vi "ELeye_V3.vi"() -> ()   [LabVIEW 2018]
uses:
  Keithley_622x_LV_8/Keithley 622x LV 8.0/Utility/Typedefs/KE622x -- Instrument Type.ctl
  Keithley_622x_LV_8/Keithley 622x LV 8.0/Typedefs/KE622x -- On Off Control.ctl
  Keithley_622x_LV_8/Keithley 622x LV 8.0/Configure/Source/Typedefs/KE622x -- Current Level.ctl
  ke236/KE236.LLB/Keith 236 Operate/Standby.vi
  <vilib>/Instr/_visa.llb/VISA Configure Serial Port (Instr).vi
  <vilib>/Utility/file.llb/Write Delimited Spreadsheet (DBL).vi
  Keithley_622x_LV_8/Keithley 622x LV 8.0/Keithley 622x.lvlib
panel:
  in  "Interline Delay (s)":dbl
  in  "SMU GPIB address":string="16"
  out "1D values":dbl[](array[numeric]) format="%.2f"
  out "1D Data ready":bool caption="1D ready"
  out "2D Data ready":bool caption="2D ready"
  in  "Filaname":string
  out "Y scale":dbl[](array[numeric]) format="%.2f"
  out "X scale":dbl[](array[numeric]) format="%.2f"
  out "2D XY array":dbl[][](array[numeric])
  out "IV 1D Graph":T1(graph)
  out "Time Trace":dbl(graph)
  in  "Sample SMU?":bool caption="SMU"
  in  "Sample Current Source?":bool caption="Source I"
  in  "Sample Gate?":bool caption="Gate V"
  out "Error SMU":errorcluster
  in  "Save":bool
  in  "Save Path":path
  in  "Compliance Current Drain":dbl=1e-06 caption="Compliance (A)" min=-0.001 max=0.001 step=1e-09 format="%#_6e"
  in  "Start VdVg Sweep":bool
  out "SMU Device Ready":bool
  in  "Initialize SMU":bool
  in  "SMU Resource":refnum<visa-resource-name> caption="SMU"
  out "Drain Device Ready":bool
  in  "Initialize Drain Source":bool
  in  "Compliance Shutoff":bool
  out "Voltage-Current 2D Graph":dbl[][](graph)
  out "Gate Device Ready":bool
  in  "Initialize Gate Generator":bool
  in  "Start IdVg Sweep":bool
  out "Error Current":errorcluster
  in  "Current Resource":refnum<visa-resource-name> caption="Current Source"
  out "Present Time":dbl caption="Time (s)"
  in  "Start Drain Sweep":bool
  out "Voltage Gate Value":dbl
  out "Voltage Drain Value":dbl
  in  "Step Voltage Drain":dbl
  in  "End Voltage Drain":dbl=-0.1
  in  "Start Voltage Drain":dbl=-0.1
  in  "Start Gate Sweep":bool
  in  "Sampling Mode":u16(ring) items=["Source V/Measure I", "Source I/Measure V"]
  in  "Start Voltage Gate":dbl=-2.0 caption="Start"
  in  "End Voltage Gate":dbl=2.0 caption="End"
  in  "Step Voltage Gate":dbl=0.1 caption="Step"
  in  "Sampling Number":u32=10 caption="Samples Number"
  in  "Start Sampling":bool
  in  "Stop Measurements":bool
  in  "Start CC Sweep":bool
  in  "Start Current Drain":dbl=1e-06 min=-0.001 max=0.001 step=1e-09 format="%#.6e"
  in  "End Current Drain":dbl=1e-06 min=-0.001 max=0.001 step=1e-09 format="%#_6e"
  in  "Step Current Drain":dbl=1e-06 min=-0.001 max=0.001 step=1e-09
  in  "Compliance Voltage Drain":dbl=10.0 caption="Compliance (V)"
  out "Current Drain Value":dbl
  out "Current Gate Value":dbl
  in  "Integration Time":dbl=100.0 caption="Int. Time (s)" format="%#_1f"
  in  "OneWay Sweep":bool caption="OneWay"
  in  "Step Delay (s)":dbl
  in  "Exit program":bool
  out "Error Gate":errorcluster
  in  "Gate resource":refnum<visa-resource-name> caption="Gate Generator"
  # "Gate (V)"
  # "Drain (V)"
  # "Drain (A)"
  # "Drain"
  # "Gate"
  # "(A)"
  # "(V)"
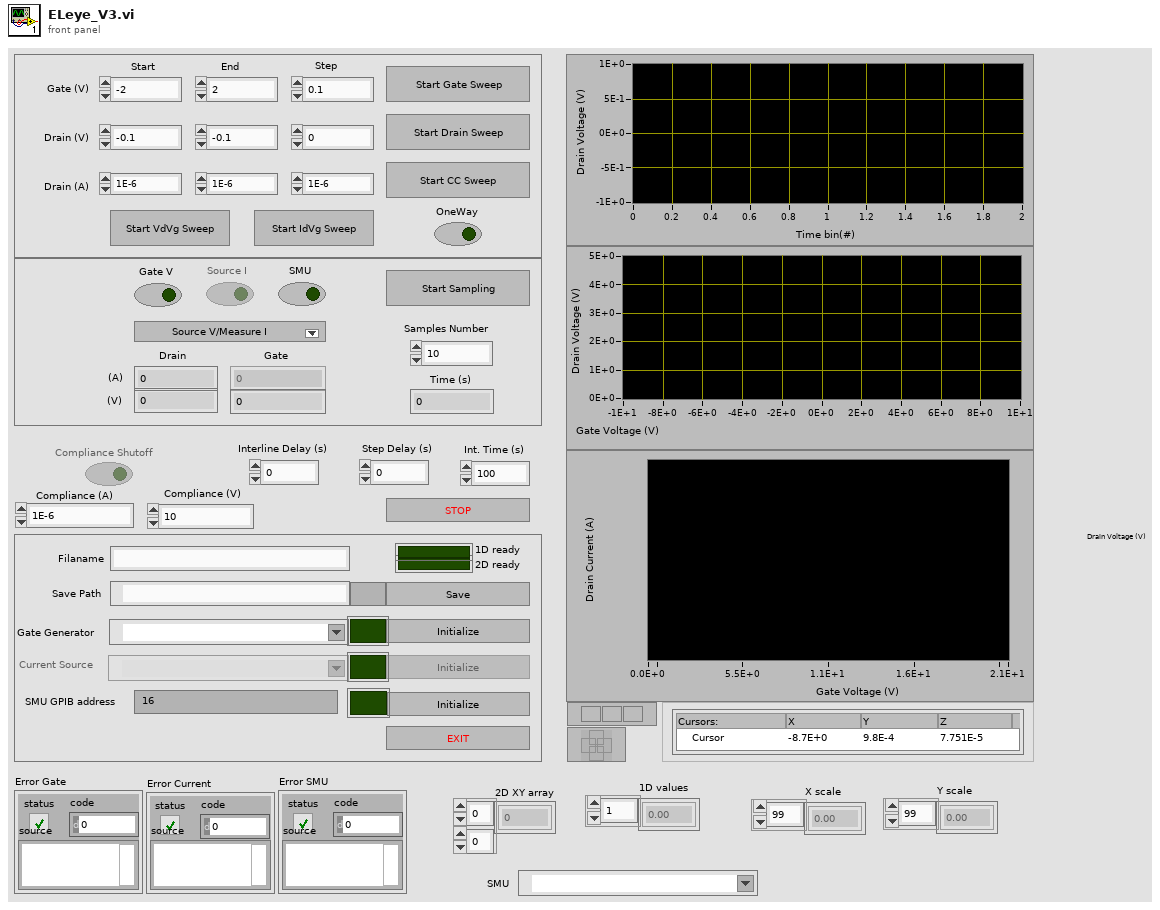
[diagram p1: front panel]
types:
  T1 = cluster{"Calibrated Array":dbl[], "Array F32":sgl[]}
  T2 = typedef "Keithley 622x.lvlib/KE622x -- On Off Control.ctl" = enum16{"Off", "On"}
  T3 = typedef "Keithley 622x.lvlib/KE622x -- Current Level.ctl" = dbl
  T4 = typedef "Keithley 622x.lvlib/KE622x -- Instrument Type.ctl" = enum16{"KE6220", "KE6221"}
  T5 = cluster{"error":bool, "code":i32, "source":string}
  T6 = cluster{"source value":string, "measure value":string, "delay value (sec)":string, "time value (sec)":string}[]
  T7 = cluster{"source value":dbl, "measure value":dbl, "delay value (sec)":dbl, "time value (sec)":dbl}[]
  T8 = cluster{"source value":dbl, "measure value":dbl, "delay value (sec)":dbl, "time value (sec)":dbl}
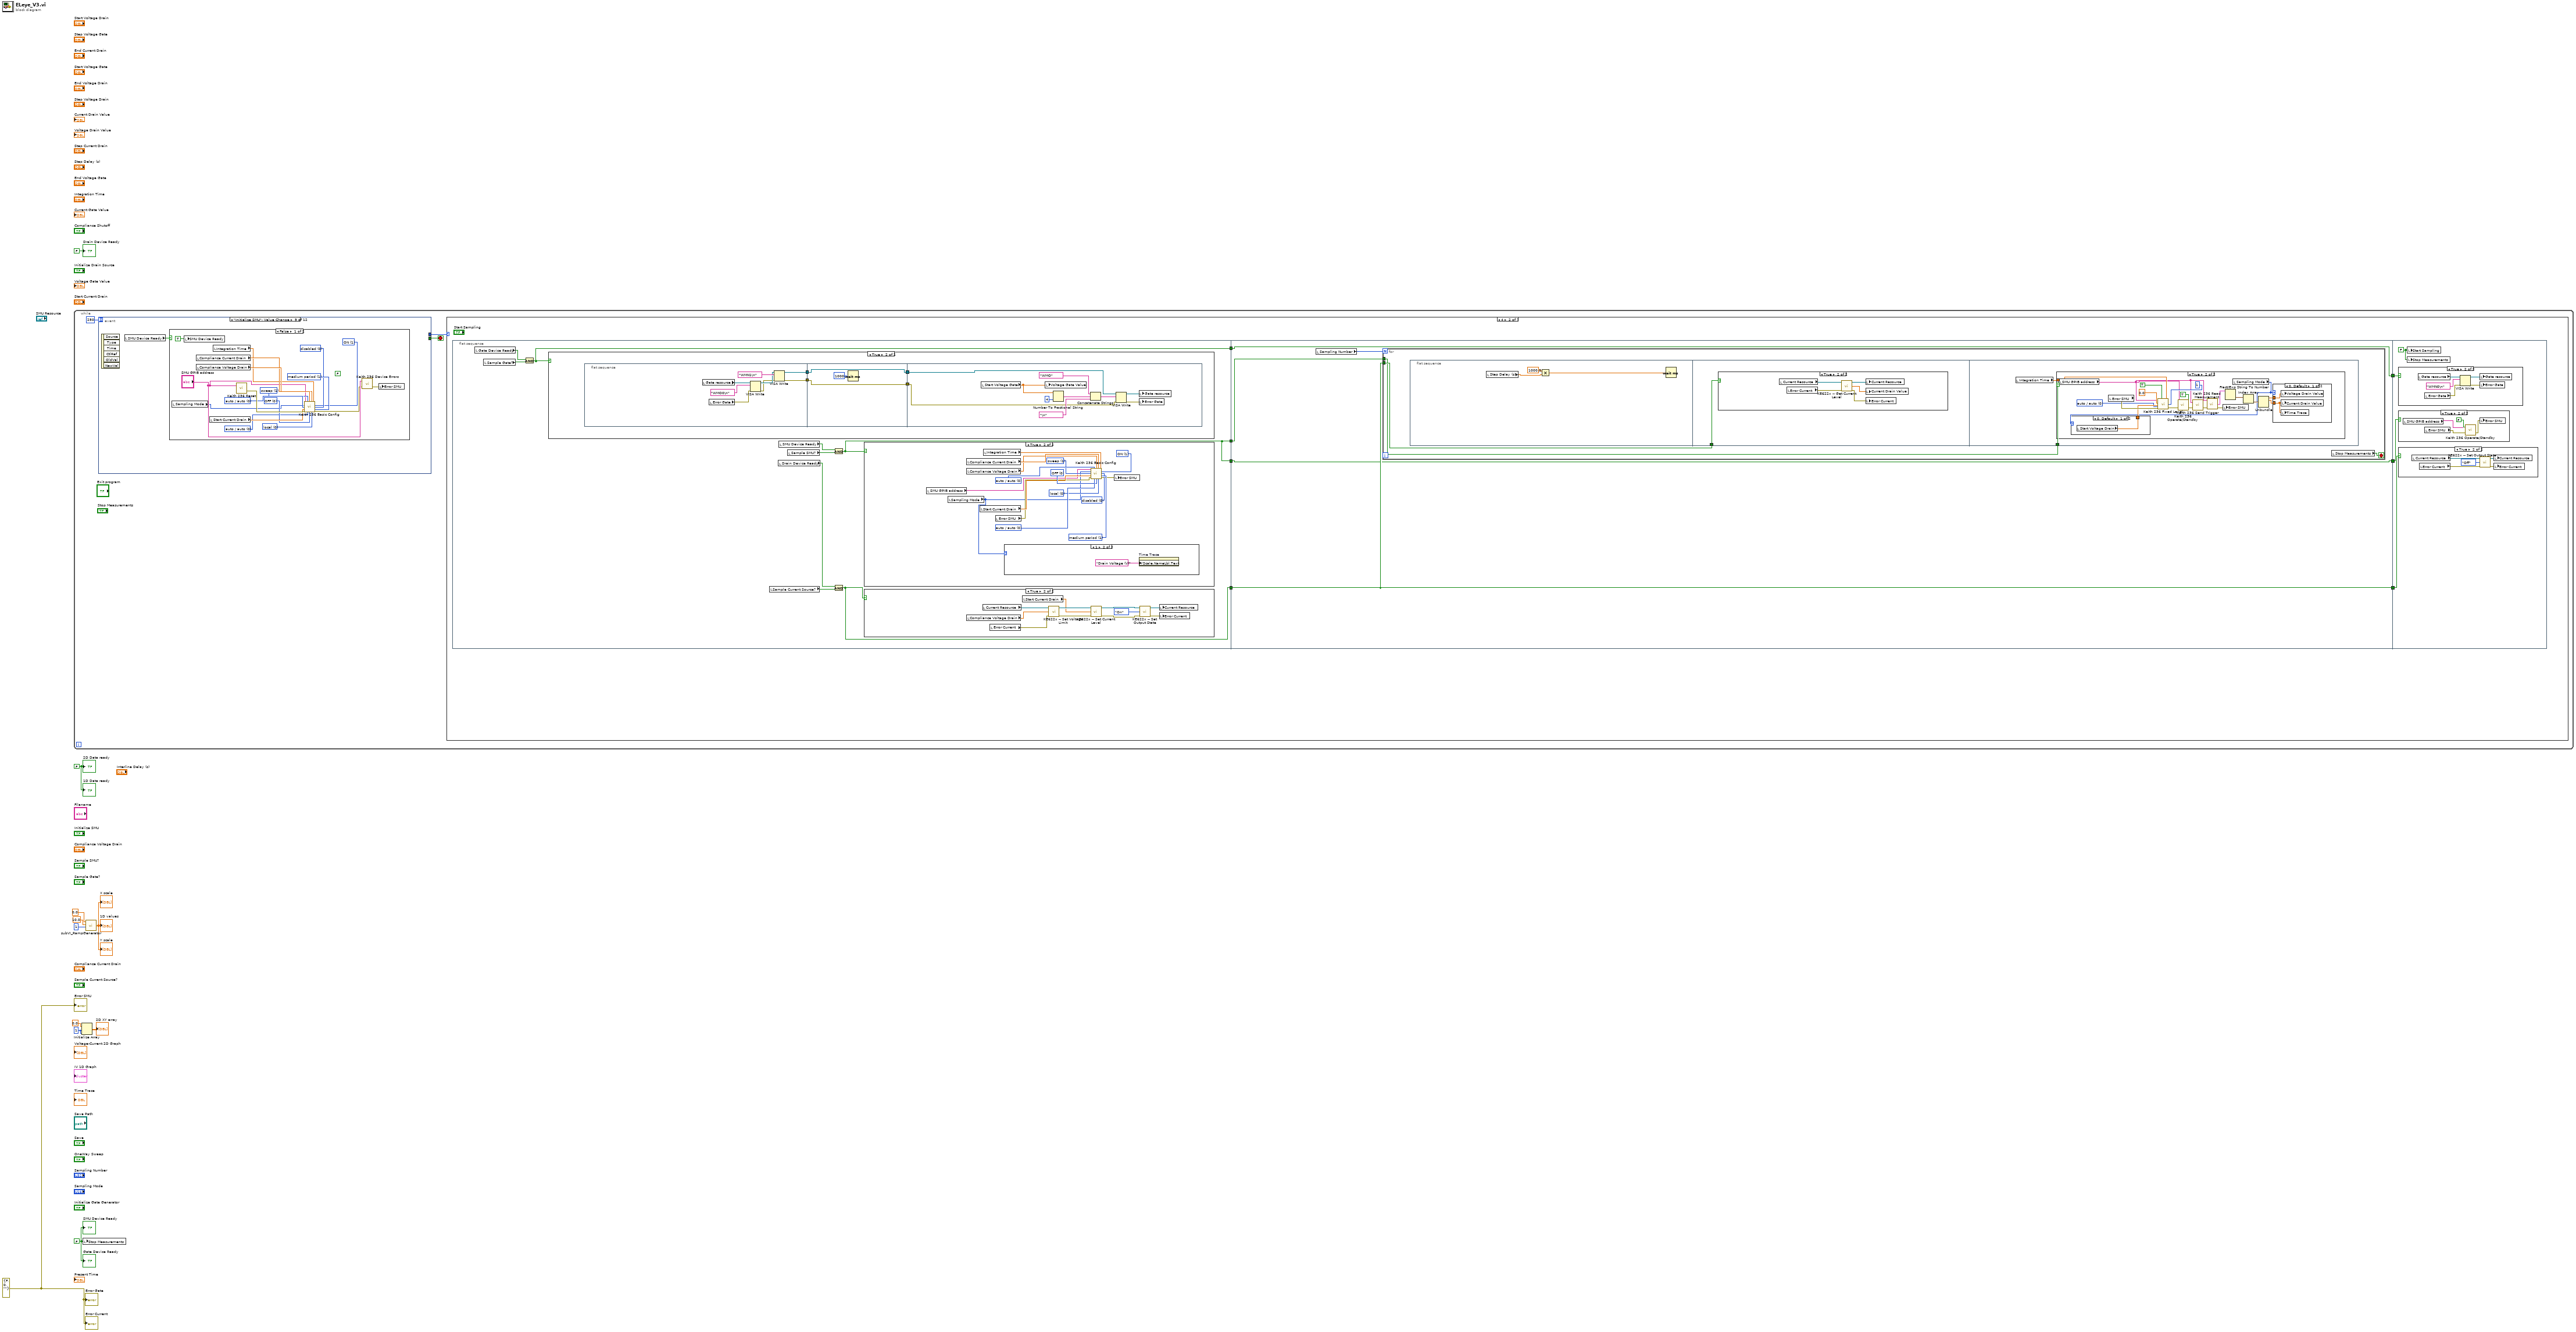
[diagram p0: block diagram]
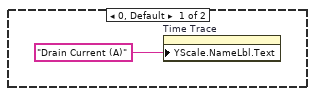
[diagram p4: hidden frame]
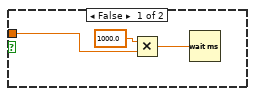
[diagram p8: hidden frame]
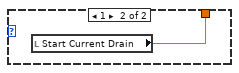
[diagram p9: hidden frame]
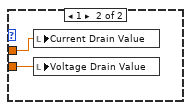
[diagram p10: hidden frame]
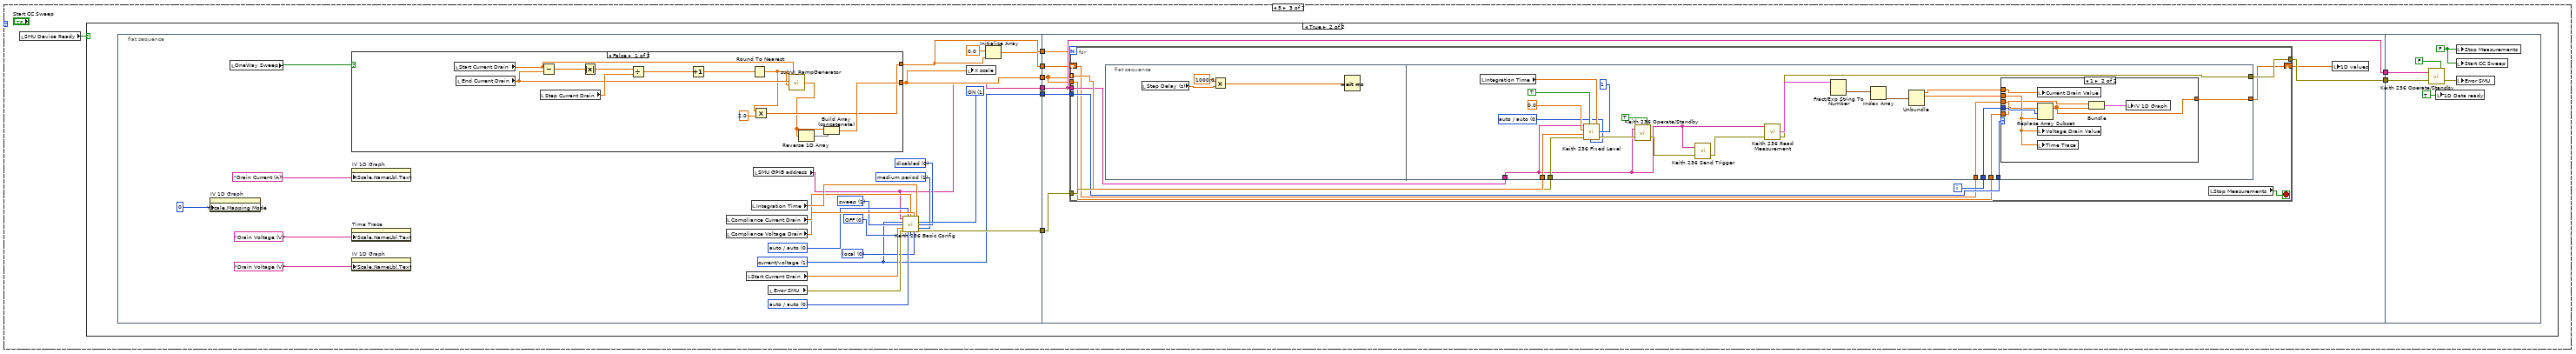
[diagram p14: hidden frame]
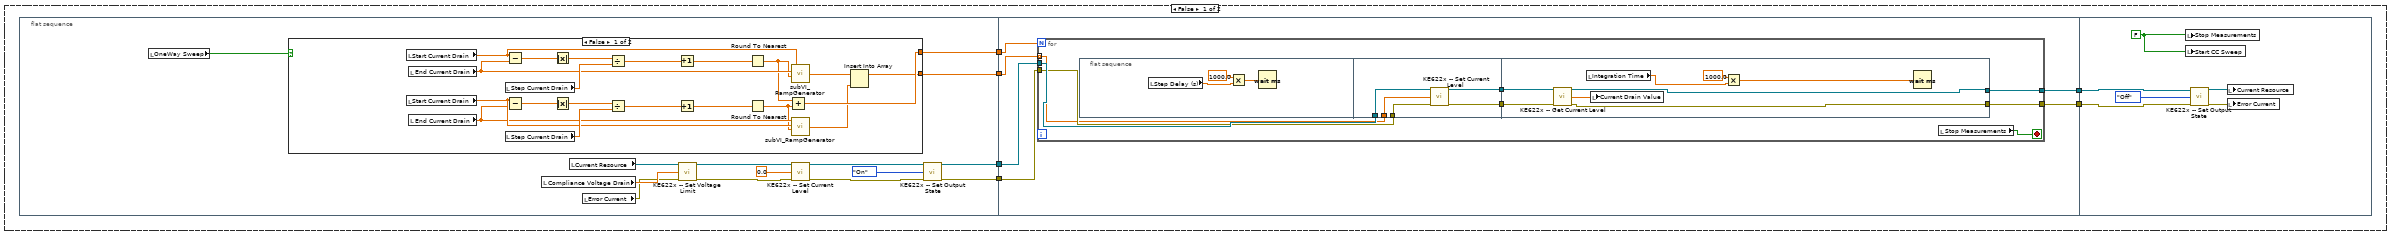
[diagram p15: hidden frame]
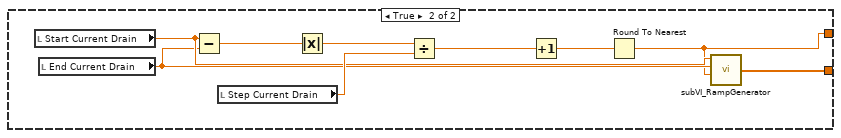
[diagram p16: hidden frame]
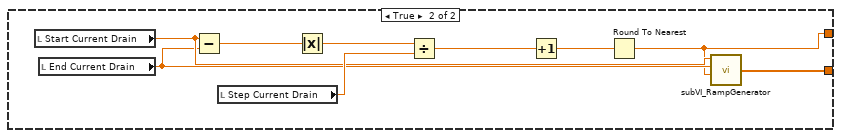
[diagram p17: hidden frame]
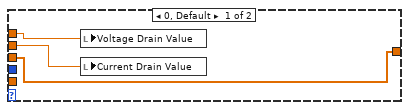
[diagram p18: hidden frame]
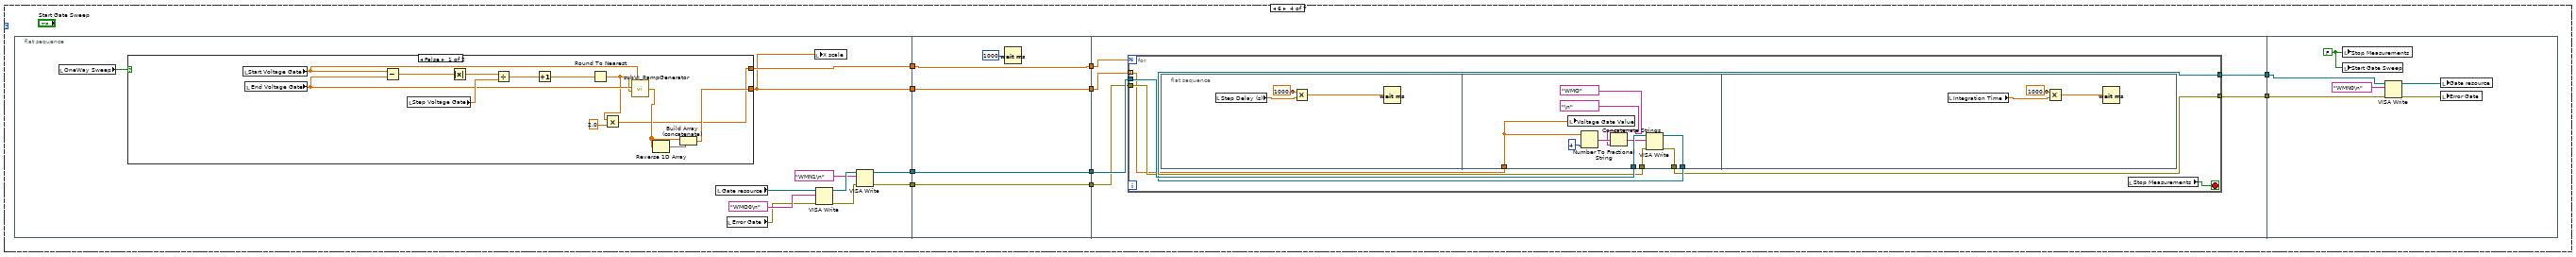
[diagram p19: hidden frame]
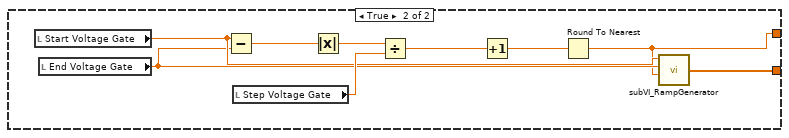
[diagram p20: hidden frame]
diagram:
  w2 = FALSE ("Data ready")
  w8 = 1 ("dimension size")
  w1 = errorcluster {"status"=FALSE, "code"=0, "source"=""} ("Error Gate")
  w10 = FALSE ("Devices Ready")
  n1 = while {
    stop <- w12 stop-if-true
    n2 = event shown="[8] \"Initialize SMU\": Value Change" {
      selector: _ -> [_ _ _ _ _ _ _ _ _ _ _ _]
      dyn-events: _ -> [_ _ _ _ _ _ _ _ _ _ _ _]
      timeout: 250 -> [_ _ _ _ _ _ _ _ _ _ _ _]
      tunnel: [_ TRUE _ _ _ _ _ _ _ _ _ _] -> w12
      tunnel: [0 _ _ _ w1024 w1030 w1033 w1037 _ w1063 w1066 _] -> w13
      event Timeout {
        n3 = event-data() -> ()  [unwired: 1 in, 3 out]
      }
      event Application Instance Close; Panel Close; "Exit program": Value Change {
        n4 = event-data() -> ()  [unwired: 1 in, 3 out]
        n5 = local read "Drain Device Ready"() -> (w976:bool)
        n6 = local read "SMU Device Ready"() -> (w975:bool)
        n7 = local read "Gate Device Ready"() -> (w977:bool)
        n8 = case shown="True" w975 {
          frame False {
          }
          frame True {
            n9 = local read "SMU GPIB address"() -> (w979:string)
            n10 = local read "Error SMU"() -> (w982:errorcluster)
            n11 = call "Keith 236 Operate/Standby.vi"("source"=FALSE, "error in"=w982, "GPIB address"=w979) -> ("error out"=w980:T5)
            n12 = local write "Error SMU"(w980) -> ()
          }
        }
        n13 = case shown="True" w977 {
          frame False {
          }
          frame True {
            n14 = local read "Gate resource"() -> (w987:refnum<visa-resource-name>)
            n15 = local read "Error Gate"() -> (w988:errorcluster)
            n16 = VISA Write(VISA resource name=w987, write buffer="WMN0\n", error in (no error)=w988) -> (VISA resource name out=w991:refnum<visa-resource-name>, error out=w990:errorcluster)  [unwired: 1 out]
            n17 = VISA Close(VISA resource name=w991, error in (no error)=w990) -> (error out=w986:errorcluster)
            n18 = local write "Error Gate"(w986) -> ()
          }
        }
        n19 = case shown="False" w976 {
          frame False {
          }
          frame True {
            n20 = local read "Current Resource"() -> (w984:refnum<visa-resource-name>)
            n21 = local read "Error Current"() -> (w985:errorcluster)
            n22 = call "Close.vi"("VISA resource name"=w984, "error in (no error)"=w985) -> ("error out"=w983:errorcluster)  [unwired: 13 in]
            n23 = local write "Error Current"(w983) -> ()
          }
        }
      }
      event "Initialize Gate Generator": Value Change {
        n24 = event-data() -> ()  [unwired: 1 in, 6 out]
        n25 = local read "Gate Device Ready"() -> (w992:bool)
        n26 = case shown="False" w992 {
          frame False {
            n27 = local write "Gate Device Ready"(TRUE ("Gate Device Ready")) -> ()
            n28 = call-poly "VISA Configure Serial Port"("VISA resource name"="Gate resource", "baud rate (9600)"=u32 115200) -> ("VISA resource name out"=w999:refnum<visa-resource-name>, "error out"=w1000:errorcluster)  [unwired: 12 in]
            n29 = VISA Open(error in (no error)=w1000, VISA resource name=w999) -> (VISA resource name=w1001:refnum<visa-resource-name>, error out=w1002:errorcluster)  [unwired: 3 in]
            n30 = VISA Write(VISA resource name=w1001, write buffer="WMN0\n", error in (no error)=w1002) -> (VISA resource name out=w995:refnum<visa-resource-name>, error out=w994:errorcluster)  [unwired: 1 out]
            n31 = local write "Gate resource"(w995) -> ()
            n32 = local write "Error Gate"(w994) -> ()
          }
          frame True {
          }
        }
      }
      event "Initialize Drain Source": Value Change {
        n33 = event-data() -> ()  [unwired: 1 in, 6 out]
        n34 = local read "Drain Device Ready"() -> (w1003:bool)
        n35 = case shown="False" w1003 {
          frame False {
            w1005 = TRUE ("Reset? (T)")
            n36 = local read "Compliance Voltage Drain"() -> (w1009:dbl)
            n37 = local write "Drain Device Ready"(w1005) -> ()
            n38 = call "Initialize.vi"("VISA resource name"="Current Resource", "Error Queue Option"=enum16{"Clear Error Queue", "Error Query"}."Clear Error Queue", "Instrument Type"=KE622x_--_Instrument_Type."KE6221", "error in (no error)"=errorcluster {"status"=FALSE, "code"=0, "source"=""}, "ID Query? (T)"=TRUE, "Reset? (T)"=w1005) -> ("VISA resource name out"=w1013:refnum<visa-resource-name>, "error out"=w1012:errorcluster)  [unwired: 8 in]
            n39 = call "KE622x -- Set Voltage Limit.vi"("Resource In"=w1013, "Voltage Limit (V)"=w1009, "error in (no error)"=w1012) -> ("Resource Out (dupl)"=w1011:refnum<visa-resource-name>, "error out"=w1010:errorcluster)  [unwired: 11 in]
            n40 = local write "Current Resource"(w1011) -> ()
            n41 = local write "Error Current"(w1010) -> ()
          }
          frame True {
          }
        }
      }
      event "Start Sampling": Value Change {
        n42 = event-data() -> ()  [unwired: 1 in, 6 out]
        n43 = local read "Sample Current Source?"() -> (w1018:bool)
        n44 = local read "Drain Device Ready"() -> (w1022:bool)
        n45 = local read "SMU Device Ready"() -> (w1023:bool)
        n46 = local read "Gate Device Ready"() -> (w1021:bool)
        n47 = local read "Sample SMU?"() -> (w1019:bool)
        n48 = local read "Sample Gate?"() -> (w1020:bool)
        n49 = Compound Arithmetic op=OR(w1020, w1019, w1018) -> (w1016:bool)
        n50 = Compound Arithmetic op=OR(w1023, w1022, w1021) -> (w1017:bool)
        n51 = And(x=w1017, y=w1016) -> (x .and. y?=w1015:bool)
        n52 = case shown="True" w1015 {
          tunnel: [0 4] -> w1024
          frame False {
          }
          frame True {
          }
        }
      }
      event "Start CC Sweep": Value Change {
        n53 = event-data() -> ()  [unwired: 1 in, 6 out]
        n54 = local read "Drain Device Ready"() -> (w1028:bool)
        n55 = local read "SMU Device Ready"() -> (w1029:bool)
        n56 = Or(x=w1028, y=w1029) -> (x .or. y?=w1027:bool)
        n57 = case shown="True" w1027 {
          tunnel: [0 5] -> w1030
          frame False {
          }
          frame True {
          }
        }
      }
      event "Start Gate Sweep": Value Change {
        n58 = event-data() -> ()  [unwired: 1 in, 6 out]
        n59 = local read "Gate Device Ready"() -> (w1034:bool)
        n60 = case shown="True" w1034 {
          tunnel: [0 6] -> w1033
          frame False {
          }
          frame True {
          }
        }
      }
      event "Start IdVg Sweep": Value Change {
        n61 = event-data() -> ()  [unwired: 1 in, 6 out]
        n62 = local read "SMU Device Ready"() -> (w1039:bool)
        n63 = local read "Gate Device Ready"() -> (w1038:bool)
        n64 = And(x=w1039, y=w1038) -> (x .and. y?=w1040:bool)
        n65 = case shown="True" w1040 {
          tunnel: [0 7] -> w1037
          frame False {
          }
          frame True {
          }
        }
      }
      event "Initialize SMU": Value Change {
        n66 = event-data() -> ()  [unwired: 1 in, 6 out]
        n67 = local read "SMU Device Ready"() -> (w1043:bool)
        n68 = case shown="False" w1043 {
          frame False {
            w1047 = u16 0 items=["auto / auto", "1 nA / 1.1 V", "10 nA / 11 V", "100 nA / 110 V", "0.001 mA / 110 V", "0.01 mA / 110 V", "0.1 mA / 110 V", "1 mA / 110 V", "10 mA / 110 V", "100 mA / 110 V"] ("compliance/\nmeasurement range (auto:0)")
            w1048 = u16 1 items=["OFF", "ON"] ("default delay (on:1)")
            w1049 = u16 0 items=["disabled", "2 readings", "4 readings", "8 readings", "16 readings", "32 readings"] ("filter (disabled:0)")
            w1050 = u16 1 items=["fast perod", "medium period", "line cycle period @ 50Hz", "line cycle period @ 60Hz"] ("integration time (medium:1)")
            w1051 = u16 0 items=["OFF", "ON"] ("suppression (off:0)")
            w1052 = u16 0 items=["local", "remote"] ("sense (local:0)")
            w1056 = u16 0 items=["auto / auto", "1 nA / 1.1 V", "10 nA / 11 V", "100 nA / 110 V", "0.001 mA / 110 V", "0.01 mA / 110 V", "0.1 mA / 110 V", "1 mA / 110 V", "10 mA / 110 V", "100 mA / 110 V"] ("source range\nI source / V source (auto:0)")
            w1058 = u16 1 items=["DC", "sweep"] ("function (DC:0)")
            (unwired) FALSE ("source")
            n69 = local read "Sampling Mode"() -> (w1044:u16)
            n70 = local write "SMU Device Ready"(TRUE ("SMU Device Ready")) -> ()
            n71 = local read "Compliance Current Drain"() -> (w1054:dbl)
            n72 = local read "Compliance Voltage Drain"() -> (w1055:dbl)
            n73 = local read "Start Current Drain"() -> (w1057:dbl)
            n74 = local read "Integration Time"() -> (w1053:dbl)
            n75 = call "Keith 236 Reset.vi"("GPIB address"="SMU GPIB address") -> ("error out"=w1059:T5)  [unwired: 1 in]
            n76 = call "Keith 236 Basic Config.vi"("GPIB address"="SMU GPIB address", "source range\nI source / V source (auto:0)"=w1056, "voltage \ncompliance level"=w1055, "current \ncompliance level"=w1054, "DC delay (sec)"=w1053, "source/measure (V/I:0)"=w1044, "default delay (on:1)"=w1048, "function (DC:0)"=w1058, "filter (disabled:0)"=w1049, "source level"=w1057, "integration time (medium:1)"=w1050, "error in"=w1059, "compliance/\nmeasurement range (auto:0)"=w1047, "suppression (off:0)"=w1051, "sense (local:0)"=w1052) -> ("error out"=w1045:T5)
            n77 = call "Keith 236 Device Errors.vi"("error in"=w1045, "GPIB address"="SMU GPIB address") -> ("error out"=w1060:T5)  [unwired: 1 out]
            n78 = local write "Error SMU"(w1060) -> ()
          }
          frame True {
          }
        }
      }
      event "Start Drain Sweep": Value Change {
        n79 = event-data() -> ()  [unwired: 1 in, 6 out]
        n80 = local read "SMU Device Ready"() -> (w1062:bool)
        n81 = case shown="True" w1062 {
          tunnel: [0 9] -> w1063
          frame False {
          }
          frame True {
          }
        }
      }
      event "Start VdVg Sweep": Value Change {
        n82 = event-data() -> ()  [unwired: 1 in, 6 out]
        n83 = local read "SMU Device Ready"() -> (w1069:bool)
        n84 = local read "Gate Device Ready"() -> (w1068:bool)
        n85 = And(x=w1069, y=w1068) -> (x .and. y?=w1067:bool)
        n86 = case shown="True" w1067 {
          tunnel: [0 10] -> w1066
          frame False {
          }
          frame True {
          }
        }
      }
      event "Save": Value Change {
        n87 = event-data() -> ()  [unwired: 1 in, 6 out]
        n88 = local read "1D Data ready"() -> (w1073:bool)
        n89 = local read "2D Data ready"() -> (w1072:bool)
        n90 = case shown="True" w1073 {
          frame False {
          }
          frame True {
            n91 = local read "Filaname"() -> (w1100:string)
            n92 = local read "Save Path"() -> (w1098:path)
            n93 = local read "1D values"() -> (w1095:dbl[])
            n94 = local read "X scale"() -> (w1096:dbl[])
            n95 = Concatenate Strings(w1100, "1DXY.dat") -> (w1097:string)
            n96 = Build Path(base path=w1098, name or relative path=w1097) -> (appended path=w1102:path)
            n97 = Build Array(w1096, w1095) -> (w1094:dbl[][])
            n98 = call-poly <vilib>:"Write Delimited Spreadsheet.vi"("file path (dialog if empty)"=w1102, "format (%.3f)"="%g", "2D data"=w1094, "append to file? (new file:F)"=FALSE, "transpose? (no:F)"=TRUE ("transpose? (F)")) -> ()  [unwired: 9 in, 2 out]
          }
        }
        n99 = case shown="True" w1072 {
          frame False {
          }
          frame True {
            w1074 = "%g" ("format (%.3f)")
            w1084 = TRUE ("transpose? (F)")
            (unwired) FALSE ("append to file? (new file:F)")
            n100 = local read "Filaname"() -> (w1083:string)
            n101 = local read "Save Path"() -> (w1075:path)
            n102 = Concatenate Strings(w1083, "Xscale.dat") -> (w1088:string)
            n103 = Concatenate Strings(w1083, "Yscale.dat") -> (w1089:string)
            n104 = local read "X scale"() -> (w1079:dbl[])
            n105 = local read "Y scale"() -> (w1078:dbl[])
            n106 = Build Path(base path=w1075, name or relative path=w1088) -> (appended path=w1086:path)
            n107 = Concatenate Strings(w1083, "2DXY.dat") -> (w1077:string)
            n108 = Build Path(base path=w1075, name or relative path=w1089) -> (appended path=w1087:path)
            n109 = local read "2D XY array"() -> (w1076:dbl[][])
            n110 = Build Path(base path=w1075, name or relative path=w1077) -> (appended path=w1085:path)
            n111 = call-poly <vilib>:"Write Delimited Spreadsheet.vi"("file path (dialog if empty)"=w1086, "format (%.3f)"=w1074, "1D data"=w1079, "append to file? (new file:F)"=FALSE, "transpose? (no:F)"=w1084) -> ()  [unwired: 9 in, 2 out]
            n112 = call-poly <vilib>:"Write Delimited Spreadsheet.vi"("file path (dialog if empty)"=w1087, "format (%.3f)"=w1074, "1D data"=w1078, "append to file? (new file:F)"=FALSE, "transpose? (no:F)"=w1084) -> ()  [unwired: 9 in, 2 out]
            n113 = call-poly <vilib>:"Write Delimited Spreadsheet.vi"("file path (dialog if empty)"=w1085, "format (%.3f)"=w1074, "2D data"=w1076, "append to file? (new file:F)"=FALSE, "transpose? (no:F)"=w1084) -> ()  [unwired: 9 in, 2 out]
          }
        }
      }
    }
    n114 = case shown="4" w13 {
      frame 0, Default {
      }
      frame 4 {
        n115 = flat-sequence {
          tunnel: [w24] -> w20
          tunnel: [w23] -> w19
          tunnel: [w22] -> w17
          tunnel: [w22] -> w15
          tunnel: [w88] -> w21
          tunnel: w20 -> [w88]
          tunnel: w19 -> [w87]
          tunnel: [w87] -> w18
          tunnel: w17 -> [w86]
          tunnel: [w85] -> w16
          tunnel: w15 -> [w85]
          tunnel: w21 -> [w134]
          tunnel: w18 -> [w133]
          tunnel: w16 -> [w132]
          frame #0 {
            n116 = local read "Gate Device Ready"() -> (w25:bool)
            n117 = local read "Sample Gate?"() -> (w28:bool)
            n118 = And(x=w25, y=w28) -> (x .and. y?=w24:bool)
            n119 = case shown="True" w24 {
              frame False {
              }
              frame True {
                n120 = flat-sequence {
                  tunnel: [w65] -> w62
                  tunnel: [w64] -> w60
                  tunnel: [w73] -> w63
                  tunnel: w62 -> [w73]
                  tunnel: [w72] -> w61
                  tunnel: w60 -> [w72]
                  tunnel: w63 -> [w78]
                  tunnel: w61 -> [w75]
                  frame #0 {
                    n121 = local read "Gate resource"() -> (w67:refnum<visa-resource-name>)
                    n122 = local read "Error Gate"() -> (w68:errorcluster)
                    n123 = VISA Write(VISA resource name=w67, write buffer="WMO0\n", error in (no error)=w68) -> (VISA resource name out=w70:refnum<visa-resource-name>, error out=w69:errorcluster)  [unwired: 1 out]
                    n124 = VISA Write(VISA resource name=w70, write buffer="WMN1\n", error in (no error)=w69) -> (VISA resource name out=w65:refnum<visa-resource-name>, error out=w64:errorcluster)  [unwired: 1 out]
                  }
                  frame #1 {
                    n125 = Wait (ms)(milliseconds to wait=u32 1000) -> ()  [unwired: 1 out]
                  }
                  frame #2 {
                    n126 = local read "Start Voltage Gate"() -> (w79:dbl)
                    n127 = local write "Voltage Gate Value"(w79) -> ()
                    n128 = Number To Fractional String(number=w79, precision (6)=i16 4) -> (F-format string=w82:string)  [unwired: 2 in]
                    n129 = Concatenate Strings("WMO" ("write buffer"), w82, "\n" ("write buffer")) -> (w80:string)
                    n130 = VISA Write(VISA resource name=w78, write buffer=w80, error in (no error)=w75) -> (VISA resource name out=w77:refnum<visa-resource-name>, error out=w76:errorcluster)  [unwired: 1 out]
                    n131 = local write "Gate resource"(w77) -> ()
                    n132 = local write "Error Gate"(w76) -> ()
                  }
                }
              }
            }
            n133 = local read "Sample Current Source?"() -> (w27:bool)
            n134 = local read "Drain Device Ready"() -> (w26:bool)
            n135 = local read "SMU Device Ready"() -> (w29:bool)
            n136 = local read "Sample SMU?"() -> (w30:bool)
            n137 = And(x=w29, y=w30) -> (x .and. y?=w22:bool)
            n138 = And(x=w26, y=w27) -> (x .and. y?=w23:bool)
            n139 = case shown="True" w22 {
              frame False {
              }
              frame True {
                w35 = u16 0 items=["disabled", "2 readings", "4 readings", "8 readings", "16 readings", "32 readings"] ("filter (disabled:0)")
                w36 = u16 1 items=["OFF", "ON"] ("default delay (on:1)")
                w46 = u16 0 items=["auto / auto", "1 nA / 1.1 V", "10 nA / 11 V", "100 nA / 110 V", "0.001 mA / 110 V", "0.01 mA / 110 V", "0.1 mA / 110 V", "1 mA / 110 V", "10 mA / 110 V", "100 mA / 110 V"] ("compliance/\nmeasurement range (auto:0)")
                w45 = u16 1 items=["fast perod", "medium period", "line cycle period @ 50Hz", "line cycle period @ 60Hz"] ("integration time (medium:1)")
                w44 = u16 0 items=["OFF", "ON"] ("suppression (off:0)")
                w43 = u16 0 items=["local", "remote"] ("sense (local:0)")
                w39 = u16 0 items=["auto / auto", "1 nA / 1.1 V", "10 nA / 11 V", "100 nA / 110 V", "0.001 mA / 110 V", "0.01 mA / 110 V", "0.1 mA / 110 V", "1 mA / 110 V", "10 mA / 110 V", "100 mA / 110 V"] ("source range\nI source / V source (auto:0)")
                w37 = u16 1 items=["DC", "sweep"] ("function (DC:0)")
                n140 = local read "SMU GPIB address"() -> (w31:string)
                n141 = local read "Sampling Mode"() -> (w32:u16)
                n142 = local read "Compliance Current Drain"() -> (w41:dbl)
                n143 = local read "Compliance Voltage Drain"() -> (w40:dbl)
                n144 = local read "Start Current Drain"() -> (w38:dbl)
                n145 = local read "Integration Time"() -> (w42:dbl)
                n146 = local read "Error SMU"() -> (w34:errorcluster)
                n147 = case shown="1" w32 {
                  frame 0, Default {
                    n148 = property on="Time Trace" class="WFChart (strict)"("YScale.NameLbl.Text"="Drain Current (A)" ("Y Scale.Name Label.Text")) -> ()  [unwired: 2 in, 2 out]
                  }
                  frame 1 {
                    n149 = property on="Time Trace" class="WFChart (strict)"("YScale.NameLbl.Text"="Drain Voltage (V)" ("Y Scale.Name Label.Text")) -> ()  [unwired: 2 in, 2 out]
                  }
                }
                n150 = call "Keith 236 Basic Config.vi"("GPIB address"=w31, "source range\nI source / V source (auto:0)"=w39, "voltage \ncompliance level"=w40, "current \ncompliance level"=w41, "DC delay (sec)"=w42, "source/measure (V/I:0)"=w32, "default delay (on:1)"=w36, "function (DC:0)"=w37, "filter (disabled:0)"=w35, "source level"=w38, "integration time (medium:1)"=w45, "error in"=w34, "compliance/\nmeasurement range (auto:0)"=w46, "suppression (off:0)"=w44, "sense (local:0)"=w43) -> ("error out"=w33:T5)
                n151 = local write "Error SMU"(w33) -> ()
              }
            }
            n152 = case shown="True" w23 {
              frame False {
              }
              frame True {
                n153 = local read "Compliance Voltage Drain"() -> (w55:dbl)
                n154 = local read "Current Resource"() -> (w56:refnum<visa-resource-name>)
                n155 = local read "Error Current"() -> (w58:errorcluster)
                n156 = local read "Start Current Drain"() -> (w51:dbl)
                n157 = call "KE622x -- Set Voltage Limit.vi"("Resource In"=w56, "Voltage Limit (V)"=w55, "error in (no error)"=w58) -> ("Resource Out (dupl)"=w57:refnum<visa-resource-name>, "error out"=w59:errorcluster)  [unwired: 11 in]
                n158 = call "KE622x -- Set Current Level.vi"("Resource In"=w57, "Current Level (A) In"=w51, "error in (no error)"=w59) -> ("Resource Out (dupl)"=w53:refnum<visa-resource-name>, "error out"=w54:errorcluster)  [unwired: 10 in, 1 out]
                n159 = call "KE622x -- Set Output State.vi"("Resource In"=w53, "Output State"=KE622x_--_On_Off_Control."On", "error in (no error)"=w54) -> ("Resource Out (dupl)"=w50:refnum<visa-resource-name>, "error out"=w49:errorcluster)  [unwired: 11 in]
                n160 = local write "Current Resource"(w50) -> ()
                n161 = local write "Error Current"(w49) -> ()
              }
            }
          }
          frame #1 {
            n162 = local read "Sampling Number"() -> (w89:u32)
            n163 = for {
              N: w89 -> [_]
              tunnel: w87 -> [w91]
              tunnel: w86 -> [w90]
              stop <- w92 stop-if-true
              n164 = flat-sequence {
                tunnel: w91 -> [w96]
                tunnel: w90 -> [w103]
                frame #0 {
                  n165 = local read "Step Delay (s)"() -> (w95:dbl)
                  n166 = Multiply(x=1000.0, y=w95) -> (x*y=w93:dbl)
                  n167 = Wait (ms)(milliseconds to wait=w93) -> ()  [unwired: 1 out]
                }
                frame #1 {
                  n168 = case shown="True" w96 {
                    frame False {
                    }
                    frame True {
                      n169 = local read "Current Resource"() -> (w98:refnum<visa-resource-name>)
                      n170 = local read "Error Current"() -> (w97:errorcluster)
                      n171 = call "KE622x -- Get Current Level.vi"("Resource In"=w98, "error in (no error)"=w97) -> ("Resource Out (dupl)"=w99:refnum<visa-resource-name>, "Current Level (A)"=w101:T3, "error out"=w100:errorcluster)  [unwired: 11 in]
                      n172 = local write "Current Resource"(w99) -> ()
                      n173 = local write "Current Drain Value"(w101) -> ()
                      n174 = local write "Error Current"(w100) -> ()
                    }
                  }
                }
                frame #2 {
                  n175 = local read "Integration Time"() -> (w102:dbl)
                  n176 = case shown="True" w103 {
                    tunnel: w102 -> [w105 w120]
                    frame False {
                      n177 = Multiply(x=1000.0, y=w105) -> (x*y=w106:dbl)
                      n178 = Wait (ms)(milliseconds to wait=w106) -> ()  [unwired: 1 out]
                    }
                    frame True {
                      w112 = u16 0 items=["auto / auto", "1 nA / 1.1 V", "10 nA / 11 V", "100 nA / 110 V", "0.001 mA / 110 V", "0.01 mA / 110 V", "0.1 mA / 110 V", "1 mA / 110 V", "10 mA / 110 V", "100 mA / 110 V"] ("source range\nI source / V source (auto:0)")
                      n179 = local read "SMU GPIB address"() -> (w108:string)
                      n180 = local read "Error SMU"() -> (w124:errorcluster)
                      n181 = local read "Sampling Mode"() -> (w111:u16)
                      n182 = case shown="0, Default" w111 {
                        tunnel: [w126 w127] -> w122
                        frame 0, Default {
                          n183 = local read "Start Voltage Drain"() -> (w126:dbl)
                        }
                        frame 1 {
                          n184 = local read "Start Current Drain"() -> (w127:dbl)
                        }
                      }
                      n185 = call "Keith 236 Fixed Level.vi"("GPIB address"=w108, "create/append"=TRUE, "bias level"=0.0, "sweep level"=w122, "source range\nI source / V source (auto:0)"=w112, "error in"=w124, "delay (sec)"=w120, "count"=1) -> ("error out"=w107:T5)
                      n186 = call "Keith 236 Operate/Standby.vi"("source"=TRUE, "error in"=w107, "GPIB address"=w108) -> ("error out"=w110:T5)
                      n187 = call "Keith 236 Send Trigger.vi"("GPIB address"=w108, "error in"=w110) -> ("error out"=w109:T5)
                      n188 = call "Keith 236 Read Measurement.vi"("error in"=w109, "GPIB address"=w108) -> ("error out"=w119:T5, "display"=w117:T6)  [unwired: 2 out]
                      n189 = local write "Error SMU"(w119) -> ()
                      n190 = Fract/Exp String To Number(string=w117) -> (number=w116:T7)  [unwired: 3 in, 1 out]
                      n191 = Index Array(array=w116) -> (element=w115:T8)  [unwired: 1 in]
                      n192 = Unbundle(w115) -> ("source value"=w114:dbl, "measure value"=w113:dbl)  [unwired: 2 out]
                      n193 = case shown="0, Default" w111 {
                        tunnel: w114 -> [w129 w131]
                        tunnel: w113 -> [w128 w130]
                        frame 0, Default {
                          n194 = local write "Voltage Drain Value"(w129) -> ()
                          n195 = local write "Current Drain Value"(w128) -> ()
                          n196 = local write "Time Trace"(w128) -> ()
                        }
                        frame 1 {
                          n197 = local write "Current Drain Value"(w131) -> ()
                          n198 = local write "Voltage Drain Value"(w130) -> ()
                        }
                      }
                    }
                  }
                }
              }
              n199 = local read "Stop Measurements"() -> (w92:bool)
            }
          }
          frame #2 {
            w135 = FALSE ("Stop Measurements")
            n200 = case shown="True" w134 {
              frame False {
              }
              frame True {
                n201 = local read "Gate resource"() -> (w146:refnum<visa-resource-name>)
                n202 = local read "Error Gate"() -> (w145:errorcluster)
                n203 = VISA Write(VISA resource name=w146, write buffer="WMN0\n", error in (no error)=w145) -> (VISA resource name out=w148:refnum<visa-resource-name>, error out=w149:errorcluster)  [unwired: 1 out]
                n204 = local write "Gate resource"(w148) -> ()
                n205 = local write "Error Gate"(w149) -> ()
              }
            }
            n206 = case shown="True" w132 {
              frame False {
              }
              frame True {
                n207 = local read "SMU GPIB address"() -> (w136:string)
                n208 = local read "Error SMU"() -> (w138:errorcluster)
                n209 = call "Keith 236 Operate/Standby.vi"("source"=FALSE, "error in"=w138, "GPIB address"=w136) -> ("error out"=w139:T5)
                n210 = local write "Error SMU"(w139) -> ()
              }
            }
            n211 = case shown="True" w133 {
              frame False {
              }
              frame True {
                n212 = local read "Current Resource"() -> (w140:refnum<visa-resource-name>)
                n213 = local read "Error Current"() -> (w141:errorcluster)
                n214 = call "KE622x -- Set Output State.vi"("Resource In"=w140, "Output State"=KE622x_--_On_Off_Control."Off", "error in (no error)"=w141) -> ("Resource Out (dupl)"=w142:refnum<visa-resource-name>, "error out"=w143:errorcluster)  [unwired: 11 in]
                n215 = local write "Current Resource"(w142) -> ()
                n216 = local write "Error Current"(w143) -> ()
              }
            }
            n217 = local write "Start Sampling"(w135) -> ()
            n218 = local write "Stop Measurements"(w135) -> ()
          }
        }
      }
      frame 5 {
        n219 = local read "SMU Device Ready"() -> (w150:bool)
        n220 = case shown="True" w150 {
          frame False {
            n221 = flat-sequence {
              tunnel: [w159] -> w156
              tunnel: [w158] -> w155
              tunnel: [w169] -> w154
              tunnel: [w157] -> w151
              tunnel: w156 -> [w205]
              tunnel: w155 -> [w204]
              tunnel: [w203] -> w153
              tunnel: [w202] -> w152
              tunnel: w154 -> [w201]
              tunnel: w151 -> [w200]
              tunnel: w153 -> [w232]
              tunnel: w152 -> [w231]
              frame #0 {
                n222 = local read "OneWay Sweep"() -> (w170:bool)
                n223 = case shown="False" w170 {
                  tunnel: [w177 w193] -> w169
                  tunnel: [w180 w191] -> w157
                  frame False {
                    n224 = local read "Start Current Drain"() -> (w188:dbl)
                    n225 = local read "Start Current Drain"() -> (w176:dbl)
                    n226 = local read "End Current Drain"() -> (w187:dbl)
                    n227 = local read "End Current Drain"() -> (w175:dbl)
                    n228 = local read "Step Current Drain"() -> (w189:dbl)
                    n229 = local read "Step Current Drain"() -> (w182:dbl)
                    n230 = Subtract(x=w188, y=w187) -> (x-y=w186:dbl)
                    n231 = Subtract(x=w176, y=w175) -> (x-y=w183:dbl)
                    n232 = Absolute Value(x=w186) -> (abs(x)=w185:dbl)
                    n233 = Absolute Value(x=w183) -> (abs(x)=w184:dbl)
                    n234 = Divide(x=w185, y=w189) -> (x/y=w190:dbl)
                    n235 = Divide(x=w184, y=w182) -> (x/y=w181:dbl)
                    n236 = Increment(x=w190) -> (x+1=w174:dbl)
                    n237 = Increment(x=w181) -> (x+1=w172:dbl)
                    n238 = Round To Nearest(number=w174) -> (nearest integer value=w173:dbl)
                    n239 = Round To Nearest(number=w172) -> (nearest integer value=w171:dbl)
                    n240 = Add(x=w173, y=w171) -> (x+y=w180:dbl)
                    n241 = call "subVI_RampGenerator.vi"("Number of Positions"=w173, "End  (um)"=w187, "Start  (um)"=w188) -> ("Array"=w179:dbl[])  [unwired: 1 in]
                    n242 = call "subVI_RampGenerator.vi"("Number of Positions"=w171, "End  (um)"=w176, "Start  (um)"=w175) -> ("Array"=w178:dbl[])  [unwired: 1 in]
                    n243 = Insert Into Array(array=w179, new element=w178) -> (w177:dbl[])  [unwired: 1 in]
                  }
                  frame True {
                    n244 = local read "Start Current Drain"() -> (w197:dbl)
                    n245 = local read "End Current Drain"() -> (w196:dbl)
                    n246 = Subtract(x=w197, y=w196) -> (x-y=w195:dbl)
                    n247 = local read "Step Current Drain"() -> (w198:dbl)
                    n248 = Absolute Value(x=w195) -> (abs(x)=w194:dbl)
                    n249 = Divide(x=w194, y=w198) -> (x/y=w199:dbl)
                    n250 = Increment(x=w199) -> (x+1=w192:dbl)
                    n251 = Round To Nearest(number=w192) -> (nearest integer value=w191:dbl)
                    n252 = call "subVI_RampGenerator.vi"("Number of Positions"=w191, "End  (um)"=w196, "Start  (um)"=w197) -> ("Array"=w193:dbl[])  [unwired: 1 in]
                  }
                }
                n253 = local read "Compliance Voltage Drain"() -> (w166:dbl)
                n254 = local read "Current Resource"() -> (w165:refnum<visa-resource-name>)
                n255 = local read "Error Current"() -> (w163:errorcluster)
                n256 = call "KE622x -- Set Voltage Limit.vi"("Resource In"=w165, "Voltage Limit (V)"=w166, "error in (no error)"=w163) -> ("Resource Out (dupl)"=w164:refnum<visa-resource-name>, "error out"=w162:errorcluster)  [unwired: 11 in]
                n257 = call "KE622x -- Set Current Level.vi"("Resource In"=w164, "Current Level (A) In"=T3 0.0, "error in (no error)"=w162) -> ("Resource Out (dupl)"=w168:refnum<visa-resource-name>, "error out"=w167:errorcluster)  [unwired: 10 in, 1 out]
                n258 = call "KE622x -- Set Output State.vi"("Resource In"=w168, "Output State"=KE622x_--_On_Off_Control."On", "error in (no error)"=w167) -> ("Resource Out (dupl)"=w159:refnum<visa-resource-name>, "error out"=w158:errorcluster)  [unwired: 11 in]
              }
              frame #1 {
                n259 = for {
                  N: w200 -> [_]
                  tunnel: w205 -> [w213]
                  tunnel: w204 -> [w212]
                  tunnel: [w207] -> w203
                  tunnel: [w206] -> w202
                  tunnel: w201 -> [w211] mode=indexing
                  stop <- w210 stop-if-true
                  n260 = flat-sequence {
                    tunnel: w213 -> [w220]
                    tunnel: w212 -> [w219]
                    tunnel: w211 -> [w221]
                    tunnel: [w218] -> w209
                    tunnel: [w217] -> w208
                    tunnel: w209 -> [w226]
                    tunnel: w208 -> [w225]
                    tunnel: [w224] -> w207
                    tunnel: [w223] -> w206
                    frame #0 {
                      n261 = local read "Step Delay (s)"() -> (w214:dbl)
                      n262 = Multiply(x=1000.0, y=w214) -> (x*y=w216:dbl)
                      n263 = Wait (ms)(milliseconds to wait=w216) -> ()  [unwired: 1 out]
                    }
                    frame #1 {
                      n264 = call "KE622x -- Set Current Level.vi"("Resource In"=w220, "Current Level (A) In"=w221, "error in (no error)"=w219) -> ("Resource Out (dupl)"=w217:refnum<visa-resource-name>, "error out"=w218:errorcluster)  [unwired: 10 in, 1 out]
                    }
                    frame #2 {
                      n265 = call "KE622x -- Get Current Level.vi"("Resource In"=w225, "error in (no error)"=w226) -> ("Resource Out (dupl)"=w224:refnum<visa-resource-name>, "Current Level (A)"=w222:T3, "error out"=w223:errorcluster)  [unwired: 11 in]
                      n266 = local read "Integration Time"() -> (w229:dbl)
                      n267 = local write "Current Drain Value"(w222) -> ()
                      n268 = Multiply(x=1000.0, y=w229) -> (x*y=w227:dbl)
                      n269 = Wait (ms)(milliseconds to wait=w227) -> ()  [unwired: 1 out]
                    }
                  }
                  n270 = local read "Stop Measurements"() -> (w210:bool)
                }
              }
              frame #2 {
                w230 = FALSE ("Stop Measurements")
                n271 = local write "Stop Measurements"(w230) -> ()
                n272 = local write "Start CC Sweep"(w230) -> ()
                n273 = call "KE622x -- Set Output State.vi"("Resource In"=w232, "Output State"=KE622x_--_On_Off_Control."Off", "error in (no error)"=w231) -> ("Resource Out (dupl)"=w235:refnum<visa-resource-name>, "error out"=w234:errorcluster)  [unwired: 11 in]
                n274 = local write "Current Resource"(w235) -> ()
                n275 = local write "Error Current"(w234) -> ()
              }
            }
          }
          frame True {
            n276 = flat-sequence {
              tunnel: [w245] -> w243
              tunnel: [w244] -> w242
              tunnel: [w254] -> w241
              tunnel: [w253] -> w240
              tunnel: [w250] -> w237
              tunnel: [w249] -> w236
              tunnel: w243 -> [w292]
              tunnel: [w298] -> w239
              tunnel: [w297] -> w238
              tunnel: w242 -> [w297]
              tunnel: w241 -> [w296]
              tunnel: w240 -> [w295]
              tunnel: w237 -> [w294]
              tunnel: w236 -> [w293]
              tunnel: w239 -> [w348]
              tunnel: w238 -> [w347]
              frame #0 {
                w253 = u16 1 items=["voltage/current", "current/voltage"] ("source/measure (V/I:0)")
                w259 = u16 0 items=["disabled", "2 readings", "4 readings", "8 readings", "16 readings", "32 readings"] ("filter (disabled:0)")
                w261 = u16 1 items=["OFF", "ON"] ("default delay (on:1)")
                w257 = u16 0 items=["auto / auto", "1 nA / 1.1 V", "10 nA / 11 V", "100 nA / 110 V", "0.001 mA / 110 V", "0.01 mA / 110 V", "0.1 mA / 110 V", "1 mA / 110 V", "10 mA / 110 V", "100 mA / 110 V"] ("compliance/\nmeasurement range (auto:0)")
                w258 = u16 1 items=["fast perod", "medium period", "line cycle period @ 50Hz", "line cycle period @ 60Hz"] ("integration time (medium:1)")
                w256 = u16 0 items=["OFF", "ON"] ("suppression (off:0)")
                w255 = u16 0 items=["local", "remote"] ("sense (local:0)")
                w262 = u16 0 items=["auto / auto", "1 nA / 1.1 V", "10 nA / 11 V", "100 nA / 110 V", "0.001 mA / 110 V", "0.01 mA / 110 V", "0.1 mA / 110 V", "1 mA / 110 V", "10 mA / 110 V", "100 mA / 110 V"] ("source range\nI source / V source (auto:0)")
                w260 = u16 1 items=["DC", "sweep"] ("function (DC:0)")
                n277 = property on="IV 1D Graph" class="XYGraph (strict)"("YScale.Mapping Mode"=u8 0 ("Y Scale.Mapping Mode")) -> ()  [unwired: 2 in, 2 out]
                n278 = local read "OneWay Sweep"() -> (w268:bool)
                n279 = case shown="False" w268 {
                  tunnel: [w272 w284] -> w245
                  tunnel: [w271 w282] -> w250
                  frame False {
                    n280 = local read "Start Current Drain"() -> (w279:dbl)
                    n281 = local read "End Current Drain"() -> (w278:dbl)
                    n282 = local read "Step Current Drain"() -> (w280:dbl)
                    n283 = Subtract(x=w279, y=w278) -> (x-y=w277:dbl)
                    n284 = Absolute Value(x=w277) -> (abs(x)=w276:dbl)
                    n285 = Divide(x=w276, y=w280) -> (x/y=w281:dbl)
                    n286 = Increment(x=w281) -> (x+1=w275:dbl)
                    n287 = Round To Nearest(number=w275) -> (nearest integer value=w270:dbl)
                    n288 = Multiply(x=w270, y=2.0) -> (x*y=w271:dbl)
                    n289 = call "subVI_RampGenerator.vi"("Number of Positions"=w270, "End  (um)"=w278, "Start  (um)"=w279) -> ("Array"=w269:dbl[])  [unwired: 1 in]
                    n290 = Reverse 1D Array(array=w269) -> (reversed array=w273:dbl[])
                    n291 = Build Array (concatenate)(w269, w273) -> (w272:dbl[])
                  }
                  frame True {
                    n292 = local read "Start Current Drain"() -> (w288:dbl)
                    n293 = local read "End Current Drain"() -> (w287:dbl)
                    n294 = Subtract(x=w288, y=w287) -> (x-y=w286:dbl)
                    n295 = local read "Step Current Drain"() -> (w289:dbl)
                    n296 = Absolute Value(x=w286) -> (abs(x)=w285:dbl)
                    n297 = Divide(x=w285, y=w289) -> (x/y=w290:dbl)
                    n298 = Increment(x=w290) -> (x+1=w283:dbl)
                    n299 = Round To Nearest(number=w283) -> (nearest integer value=w282:dbl)
                    n300 = call "subVI_RampGenerator.vi"("Number of Positions"=w282, "End  (um)"=w287, "Start  (um)"=w288) -> ("Array"=w284:dbl[])  [unwired: 1 in]
                  }
                }
                n301 = property on="IV 1D Graph" class="XYGraph (strict)"("XScale.NameLbl.Text"="Drain Current (A)" ("Y Scale.Name Label.Text")) -> ()  [unwired: 2 in, 2 out]
                n302 = property on="Time Trace" class="WFChart (strict)"("YScale.NameLbl.Text"="Drain Voltage (V)" ("Y Scale.Name Label.Text")) -> ()  [unwired: 2 in, 2 out]
                n303 = property on="IV 1D Graph" class="XYGraph (strict)"("YScale.NameLbl.Text"="Drain Voltage (V)" ("Y Scale.Name Label.Text")) -> ()  [unwired: 2 in, 2 out]
                n304 = local read "Compliance Current Drain"() -> (w266:dbl)
                n305 = local read "Compliance Voltage Drain"() -> (w265:dbl)
                n306 = local read "Start Current Drain"() -> (w264:dbl)
                n307 = local read "Integration Time"() -> (w267:dbl)
                n308 = local read "SMU GPIB address"() -> (w244:string)
                n309 = local read "Error SMU"() -> (w263:errorcluster)
                n310 = call "Keith 236 Basic Config.vi"("GPIB address"=w244, "source range\nI source / V source (auto:0)"=w262, "voltage \ncompliance level"=w265, "current \ncompliance level"=w266, "DC delay (sec)"=w267, "source/measure (V/I:0)"=w253, "default delay (on:1)"=w261, "function (DC:0)"=w260, "filter (disabled:0)"=w259, "source level"=w264, "integration time (medium:1)"=w258, "error in"=w263, "compliance/\nmeasurement range (auto:0)"=w257, "suppression (off:0)"=w256, "sense (local:0)"=w255) -> ("error out"=w254:T5)
                n311 = local write "X scale"(w245) -> ()
                n312 = Initialize Array(0.0, w250) -> (w249:dbl[])
              }
              frame #1 {
                n313 = for {
                  N: w294 -> [_]
                  tunnel: w292 -> [w307] mode=indexing
                  tunnel: [w306] -> w298
                  tunnel: w297 -> [w305]
                  tunnel: w296 -> [w304]
                  tunnel: w295 -> [w303]
                  shift-right: [w301] -> w291
                  shift-left: w293 -> [w300]
                  tunnel: w292 -> [w299]
                  i -> [w302]
                  stop <- w308 stop-if-true
                  n314 = flat-sequence {
                    tunnel: w307 -> [w324]
                    tunnel: [w322] -> w306
                    tunnel: w305 -> [w312]
                    tunnel: w304 -> [w321]
                    tunnel: w303 -> [w320]
                    tunnel: w302 -> [w318]
                    tunnel: [w317] -> w301
                    tunnel: w300 -> [w316]
                    tunnel: w299 -> [w315]
                    frame #0 {
                      n315 = local read "Step Delay (s)"() -> (w309:dbl)
                      n316 = Multiply(x=1000.0, y=w309) -> (x*y=w311:dbl)
                      n317 = Wait (ms)(milliseconds to wait=w311) -> ()  [unwired: 1 out]
                    }
                    frame #1 {
                      w319 = u16 0 items=["auto / auto", "1 nA / 1.1 V", "10 nA / 11 V", "100 nA / 110 V", "0.001 mA / 110 V", "0.01 mA / 110 V", "0.1 mA / 110 V", "1 mA / 110 V", "10 mA / 110 V", "100 mA / 110 V"] ("source range\nI source / V source (auto:0)")
                      n318 = local read "Integration Time"() -> (w323:dbl)
                      n319 = call "Keith 236 Fixed Level.vi"("GPIB address"=w312, "create/append"=TRUE, "bias level"=0.0, "sweep level"=w324, "source range\nI source / V source (auto:0)"=w319, "error in"=w321, "delay (sec)"=w323, "count"=1) -> ("error out"=w329:T5)
                      n320 = call "Keith 236 Operate/Standby.vi"("source"=TRUE, "error in"=w329, "GPIB address"=w312) -> ("error out"=w314:T5)
                      n321 = call "Keith 236 Send Trigger.vi"("GPIB address"=w312, "error in"=w314) -> ("error out"=w313:T5)
                      n322 = call "Keith 236 Read Measurement.vi"("error in"=w313, "GPIB address"=w312) -> ("error out"=w322:T5, "display"=w330:T6)  [unwired: 2 out]
                      n323 = Fract/Exp String To Number(string=w330) -> (number=w331:T7)  [unwired: 3 in, 1 out]
                      n324 = Index Array(array=w331) -> (element=w332:T8)  [unwired: 1 in]
                      n325 = Unbundle(w332) -> ("source value"=w333:dbl, "measure value"=w334:dbl)  [unwired: 2 out]
                      n326 = case shown="1" w320 {
                        tunnel: w333 -> [w337 w344]
                        tunnel: w334 -> [w336 w342]
                        tunnel: w318 -> [_ w343]
                        tunnel: [w335 w339] -> w317
                        tunnel: w316 -> [w335 w341]
                        tunnel: w315 -> [_ w340]
                        frame 0, Default {
                          n327 = local write "Voltage Drain Value"(w337) -> ()
                          n328 = local write "Current Drain Value"(w336) -> ()
                        }
                        frame 1 {
                          n329 = local write "Current Drain Value"(w344) -> ()
                          n330 = local write "Voltage Drain Value"(w342) -> ()
                          n331 = local write "Time Trace"(w342) -> ()
                          n332 = Replace Array Subset(array=w341, new element=w342, index=w343) -> (w339:dbl[])
                          n333 = Bundle("Array"=w340, w339) -> (w338:cluster{"Array":dbl[], dbl[]})  [unwired: 1 in]
                          n334 = local write "IV 1D Graph"(w338) -> ()
                        }
                      }
                    }
                  }
                  n335 = local read "Stop Measurements"() -> (w308:bool)
                }
                n336 = local write "1D values"(w291) -> ()
              }
              frame #2 {
                w346 = FALSE ("Stop Measurements")
                n337 = call "Keith 236 Operate/Standby.vi"("source"=FALSE, "error in"=w348, "GPIB address"=w347) -> ("error out"=w350:T5)
                n338 = local write "1D Data ready"(TRUE ("1D Data ready")) -> ()
                n339 = local write "Stop Measurements"(w346) -> ()
                n340 = local write "Start CC Sweep"(w346) -> ()
                n341 = local write "Error SMU"(w350) -> ()
              }
            }
          }
        }
      }
      frame 6 {
        n342 = flat-sequence {
          tunnel: [w365] -> w358
          tunnel: [w364] -> w356
          tunnel: [w361] -> w354
          tunnel: [w362] -> w352
          tunnel: w358 -> [w398]
          tunnel: [w398] -> w357
          tunnel: w356 -> [w397]
          tunnel: [w397] -> w355
          tunnel: w354 -> [w396]
          tunnel: [w396] -> w353
          tunnel: w352 -> [w395]
          tunnel: [w395] -> w351
          tunnel: w357 -> [w404]
          tunnel: w355 -> [w403]
          tunnel: [w402] -> w360
          tunnel: [w401] -> w359
          tunnel: w353 -> [w400]
          tunnel: w351 -> [w399]
          tunnel: w360 -> [w429]
          tunnel: w359 -> [w428]
          frame #0 {
            n343 = local read "OneWay Sweep"() -> (w363:bool)
            n344 = case shown="False" w363 {
              tunnel: [w374 w387] -> w361
              tunnel: [w373 w385] -> w362
              frame False {
                n345 = local read "Start Voltage Gate"() -> (w382:dbl)
                n346 = local read "End Voltage Gate"() -> (w381:dbl)
                n347 = Subtract(x=w382, y=w381) -> (x-y=w380:dbl)
                n348 = local read "Step Voltage Gate"() -> (w383:dbl)
                n349 = Absolute Value(x=w380) -> (abs(x)=w379:dbl)
                n350 = Divide(x=w379, y=w383) -> (x/y=w384:dbl)
                n351 = Increment(x=w384) -> (x+1=w378:dbl)
                n352 = Round To Nearest(number=w378) -> (nearest integer value=w372:dbl)
                n353 = Multiply(x=w372, y=2.0) -> (x*y=w373:dbl)
                n354 = call "subVI_RampGenerator.vi"("Number of Positions"=w372, "End  (um)"=w381, "Start  (um)"=w382) -> ("Array"=w375:dbl[])  [unwired: 1 in]
                n355 = Reverse 1D Array(array=w375) -> (reversed array=w376:dbl[])
                n356 = Build Array (concatenate)(w375, w376) -> (w374:dbl[])
              }
              frame True {
                n357 = local read "Start Voltage Gate"() -> (w391:dbl)
                n358 = local read "End Voltage Gate"() -> (w390:dbl)
                n359 = Subtract(x=w391, y=w390) -> (x-y=w389:dbl)
                n360 = local read "Step Voltage Gate"() -> (w392:dbl)
                n361 = Absolute Value(x=w389) -> (abs(x)=w388:dbl)
                n362 = Divide(x=w388, y=w392) -> (x/y=w393:dbl)
                n363 = Increment(x=w393) -> (x+1=w386:dbl)
                n364 = Round To Nearest(number=w386) -> (nearest integer value=w385:dbl)
                n365 = call "subVI_RampGenerator.vi"("Number of Positions"=w385, "End  (um)"=w390, "Start  (um)"=w391) -> ("Array"=w387:dbl[])  [unwired: 1 in]
              }
            }
            n366 = local read "Gate resource"() -> (w370:refnum<visa-resource-name>)
            n367 = local read "Error Gate"() -> (w369:errorcluster)
            n368 = local write "X scale"(w361) -> ()
            n369 = VISA Write(VISA resource name=w370, write buffer="WMO0\n", error in (no error)=w369) -> (VISA resource name out=w367:refnum<visa-resource-name>, error out=w368:errorcluster)  [unwired: 1 out]
            n370 = VISA Write(VISA resource name=w367, write buffer="WMN1\n", error in (no error)=w368) -> (VISA resource name out=w365:refnum<visa-resource-name>, error out=w364:errorcluster)  [unwired: 1 out]
          }
          frame #1 {
            n371 = Wait (ms)(milliseconds to wait=u32 1000) -> ()  [unwired: 1 out]
          }
          frame #2 {
            n372 = for {
              N: w399 -> [_]
              tunnel: w404 -> [w410]
              tunnel: w403 -> [w409]
              tunnel: [w408] -> w402
              tunnel: [w407] -> w401
              tunnel: w400 -> [w406] mode=indexing
              stop <- w405 stop-if-true
              n373 = flat-sequence {
                tunnel: w410 -> [w423]
                tunnel: w409 -> [w422]
                tunnel: [w421] -> w408
                tunnel: [w420] -> w407
                tunnel: w406 -> [w414]
                frame #0 {
                  n374 = local read "Step Delay (s)"() -> (w411:dbl)
                  n375 = Multiply(x=1000.0, y=w411) -> (x*y=w413:dbl)
                  n376 = Wait (ms)(milliseconds to wait=w413) -> ()  [unwired: 1 out]
                }
                frame #1 {
                  n377 = local write "Voltage Gate Value"(w414) -> ()
                  n378 = Number To Fractional String(number=w414, precision (6)=i16 4) -> (F-format string=w417:string)  [unwired: 2 in]
                  n379 = Concatenate Strings("WMO" ("write buffer"), w417, "\n" ("write buffer")) -> (w419:string)
                  n380 = VISA Write(VISA resource name=w423, write buffer=w419, error in (no error)=w422) -> (VISA resource name out=w421:refnum<visa-resource-name>, error out=w420:errorcluster)  [unwired: 1 out]
                }
                frame #2 {
                  n381 = local read "Integration Time"() -> (w426:dbl)
                  n382 = Multiply(x=1000.0, y=w426) -> (x*y=w424:dbl)
                  n383 = Wait (ms)(milliseconds to wait=w424) -> ()  [unwired: 1 out]
                }
              }
              n384 = local read "Stop Measurements"() -> (w405:bool)
            }
          }
          frame #3 {
            w427 = FALSE ("Stop Measurements")
            n385 = local write "Stop Measurements"(w427) -> ()
            n386 = local write "Start Gate Sweep"(w427) -> ()
            n387 = VISA Write(VISA resource name=w429, write buffer="WMN0\n", error in (no error)=w428) -> (VISA resource name out=w431:refnum<visa-resource-name>, error out=w430:errorcluster)  [unwired: 1 out]
            n388 = local write "Gate resource"(w431) -> ()
            n389 = local write "Error Gate"(w430) -> ()
          }
        }
      }
      frame 7 {
        n390 = flat-sequence {
          tunnel: [w478] -> w447
          tunnel: [w448] -> w446
          tunnel: [w498] -> w445
          tunnel: [w497] -> w444
          tunnel: [w473] -> w443
          tunnel: [w488] -> w442
          tunnel: [w487] -> w441
          tunnel: [w477] -> w440
          tunnel: [w474] -> w439
          tunnel: [w483] -> w434
          tunnel: [w475] -> w433
          tunnel: w447 -> [w535]
          tunnel: [w534] -> w438
          tunnel: [w533] -> w437
          tunnel: w446 -> [w533]
          tunnel: w445 -> [w532]
          tunnel: w444 -> [w531]
          tunnel: w443 -> [w530]
          tunnel: w442 -> [w529]
          tunnel: w441 -> [w528]
          tunnel: w440 -> [w527]
          tunnel: w439 -> [w526]
          tunnel: [w525] -> w436
          tunnel: [w524] -> w435
          tunnel: w434 -> [w523]
          tunnel: w433 -> [w522]
          tunnel: w438 -> [w645]
          tunnel: w437 -> [w644]
          tunnel: w436 -> [w639]
          tunnel: w435 -> [w638]
          frame #0 {
            w476 = 0.0
            w479 = "Drain Voltage (V)" ("Y Scale.Name Label.Text")
            w497 = u16 1 items=["voltage/current", "current/voltage"] ("source/measure (V/I:0)")
            w503 = u16 0 items=["disabled", "2 readings", "4 readings", "8 readings", "16 readings", "32 readings"] ("filter (disabled:0)")
            w505 = u16 1 items=["OFF", "ON"] ("default delay (on:1)")
            w501 = u16 0 items=["auto / auto", "1 nA / 1.1 V", "10 nA / 11 V", "100 nA / 110 V", "0.001 mA / 110 V", "0.01 mA / 110 V", "0.1 mA / 110 V", "1 mA / 110 V", "10 mA / 110 V", "100 mA / 110 V"] ("compliance/\nmeasurement range (auto:0)")
            w502 = u16 1 items=["fast perod", "medium period", "line cycle period @ 50Hz", "line cycle period @ 60Hz"] ("integration time (medium:1)")
            w500 = u16 0 items=["OFF", "ON"] ("suppression (off:0)")
            w499 = u16 0 items=["local", "remote"] ("sense (local:0)")
            w506 = u16 0 items=["auto / auto", "1 nA / 1.1 V", "10 nA / 11 V", "100 nA / 110 V", "0.001 mA / 110 V", "0.01 mA / 110 V", "0.1 mA / 110 V", "1 mA / 110 V", "10 mA / 110 V", "100 mA / 110 V"] ("source range\nI source / V source (auto:0)")
            w504 = u16 1 items=["DC", "sweep"] ("function (DC:0)")
            n391 = local read "Start Current Drain"() -> (w460:dbl)
            n392 = local read "End Current Drain"() -> (w459:dbl)
            n393 = local read "Start Voltage Gate"() -> (w450:dbl)
            n394 = local read "End Voltage Gate"() -> (w449:dbl)
            n395 = flat-sequence {
              tunnel: [w513] -> w488
              tunnel: [w512] -> w487
              frame #0 {
                n396 = local read "Gate resource"() -> (w516:refnum<visa-resource-name>)
                n397 = local read "Error Gate"() -> (w517:errorcluster)
                n398 = VISA Write(VISA resource name=w516, write buffer="WMO0\n", error in (no error)=w517) -> (VISA resource name out=w519:refnum<visa-resource-name>, error out=w518:errorcluster)  [unwired: 1 out]
                n399 = VISA Write(VISA resource name=w519, write buffer="WMN1\n", error in (no error)=w518) -> (VISA resource name out=w513:refnum<visa-resource-name>, error out=w512:errorcluster)  [unwired: 1 out]
              }
              frame #1 {
                n400 = Wait (ms)(milliseconds to wait=u32 1000) -> ()  [unwired: 1 out]
              }
            }
            n401 = property on="IV 1D Graph" class="XYGraph (strict)"("YScale.Mapping Mode"=u8 0 ("Y Scale.Mapping Mode")) -> ()  [unwired: 2 in, 2 out]
            n402 = property on="Voltage-Current 2D Graph" class="IntGraph (strict)"("ZScale.Mapping Mode"=u8 0 ("Y Scale.Mapping Mode")) -> ()  [unwired: 2 in, 2 out]
            n403 = local read "Step Current Drain"() -> (w458:dbl)
            n404 = local read "Step Voltage Gate"() -> (w452:dbl)
            n405 = property on="Voltage-Current 2D Graph" class="IntGraph (strict)"("ZScale.NameLbl.Text"=w479) -> ()  [unwired: 2 in, 2 out]
            n406 = property on="IV 1D Graph" class="XYGraph (strict)"("YScale.NameLbl.Text"=w479) -> ()  [unwired: 2 in, 2 out]
            n407 = property on="IV 1D Graph" class="XYGraph (strict)"("XScale.NameLbl.Text"="Gate Voltage (V)" ("Y Scale.Name Label.Text")) -> ()  [unwired: 2 in, 2 out]
            n408 = property on="Voltage-Current 2D Graph" class="IntGraph (strict)"("XScale.NameLbl.Text"="Gate Voltage (V)" ("Y Scale.Name Label.Text")) -> ()  [unwired: 2 in, 2 out]
            n409 = property on="Voltage-Current 2D Graph" class="IntGraph (strict)"("YScale.NameLbl.Text"="Drain Current (A)" ("Y Scale.Name Label.Text")) -> ()  [unwired: 2 in, 2 out]
            n410 = property on="Time Trace" class="WFChart (strict)"("YScale.NameLbl.Text"="Drain Voltage (V)" ("Y Scale.Name Label.Text")) -> ()  [unwired: 2 in, 2 out]
            n411 = Greater?(x=w459, y=w460) -> (0:w462:bool)
            n412 = Subtract(x=w460, y=w459) -> (x-y=w495:dbl)
            n413 = Greater?(x=w449, y=w450) -> (0:w455:bool)
            n414 = Subtract(x=w450, y=w449) -> (x-y=w490:dbl)
            n415 = Absolute Value(x=w495) -> (abs(x)=w494:dbl)
            n416 = Absolute Value(x=w490) -> (abs(x)=w491:dbl)
            n417 = Divide(x=w458, y=2.0) -> (x/y=w468:dbl)
            n418 = Divide(x=w452, y=2.0) -> (x/y=w466:dbl)
            n419 = Select(t=1.0, s=w462, f=-1.0) -> (s? t:f=w461:dbl)
            n420 = Select(t=1.0, s=w455, f=-1.0) -> (s? t:f=w456:dbl)
            n421 = local read "Compliance Current Drain"() -> (w510:dbl)
            n422 = local read "Compliance Voltage Drain"() -> (w509:dbl)
            n423 = Multiply(x=w461, y=w458) -> (x*y=w457:dbl)
            n424 = Subtract(x=w460, y=w468) -> (x-y=w469:dbl)
            n425 = Divide(x=w494, y=w458) -> (x/y=w496:dbl)
            n426 = Multiply(x=w456, y=w452) -> (x*y=w451:dbl)
            n427 = Subtract(x=w450, y=w466) -> (x-y=w470:dbl)
            n428 = Divide(x=w491, y=w452) -> (x/y=w489:dbl)
            n429 = local read "SMU GPIB address"() -> (w448:string)
            n430 = local read "Start Current Drain"() -> (w508:dbl)
            n431 = local read "Integration Time"() -> (w511:dbl)
            n432 = local read "Error SMU"() -> (w507:errorcluster)
            n433 = Increment(x=w496) -> (x+1=w493:dbl)
            n434 = Increment(x=w489) -> (x+1=w492:dbl)
            n435 = property on="Voltage-Current 2D Graph" class="IntGraph (strict)"("YScale.Offset"=w469, "YScale.Multiplier"=w457, "YScale.Precision"=u8 1 ("Y Scale.Display Format:Precision")) -> ()  [unwired: 2 in, 2 out]
            n436 = property on="Voltage-Current 2D Graph" class="IntGraph (strict)"("XScale.Offset"=w470, "XScale.Multiplier"=w451, "XScale.Precision"=u8 1 ("X Scale.Display Format:Precision")) -> ()  [unwired: 2 in, 2 out]
            n437 = Round To Nearest(number=w493) -> (nearest integer value=w473:dbl)
            n438 = Round To Nearest(number=w492) -> (nearest integer value=w474:dbl)
            n439 = call "Keith 236 Basic Config.vi"("GPIB address"=w448, "source range\nI source / V source (auto:0)"=w506, "voltage \ncompliance level"=w509, "current \ncompliance level"=w510, "DC delay (sec)"=w511, "source/measure (V/I:0)"=w497, "default delay (on:1)"=w505, "function (DC:0)"=w504, "filter (disabled:0)"=w503, "source level"=w508, "integration time (medium:1)"=w502, "error in"=w507, "compliance/\nmeasurement range (auto:0)"=w501, "suppression (off:0)"=w500, "sense (local:0)"=w499) -> ("error out"=w498:T5)
            n440 = call "subVI_RampGenerator.vi"("Number of Positions"=w473, "End  (um)"=w459, "Start  (um)"=w460) -> ("Array"=w478:dbl[])  [unwired: 1 in]
            n441 = call "subVI_RampGenerator.vi"("Number of Positions"=w474, "End  (um)"=w449, "Start  (um)"=w450) -> ("Array"=w477:dbl[])  [unwired: 1 in]
            n442 = local write "Y scale"(w478) -> ()
            n443 = local write "X scale"(w477) -> ()
            n444 = Initialize Array(w476, w473, w474) -> (w475:dbl[][])
            n445 = Initialize Array(w476, w474) -> (w483:dbl[])
          }
          frame #1 {
            n446 = for {
              N: w530 -> [_]
              tunnel: w535 -> [w552] mode=indexing
              tunnel: [w551] -> w534
              tunnel: w533 -> [w550]
              tunnel: w532 -> [w549]
              tunnel: w531 -> [w548]
              tunnel: w529 -> [w547]
              tunnel: w528 -> [w546]
              tunnel: w527 -> [w540]
              tunnel: w526 -> [w545]
              tunnel: [w544] -> w525
              tunnel: [w543] -> w524
              tunnel: w523 -> [w541]
              shift-right: [w536] -> w521
              shift-left: w522 -> [w537]
              i -> [w538]
              stop <- w542 stop-if-true
              n447 = for {
                N: w545 -> [_]
                tunnel: w552 -> [w575]
                tunnel: w550 -> [w573]
                tunnel: w548 -> [w571]
                shift-right: [w574] -> w551
                shift-left: w549 -> [w572]
                tunnel: w547 -> [w559]
                tunnel: w546 -> [w558]
                tunnel: w540 -> [w557] mode=indexing
                tunnel: [w569] -> w544
                tunnel: [w568] -> w543
                tunnel: [w567] -> w542
                tunnel: w540 -> [w565]
                shift-right: [w564] -> w539
                shift-left: w541 -> [w566]
                tunnel: w538 -> [w563]
                shift-right: [w560] -> w536
                shift-left: w537 -> [w561]
                i -> [w562]
                stop <- w567 stop-if-true
                n448 = flat-sequence {
                  tunnel: w559 -> [w583]
                  tunnel: w558 -> [w582]
                  tunnel: w557 -> [w581]
                  tunnel: [w580] -> w555
                  tunnel: [w579] -> w553
                  tunnel: w575 -> [w607]
                  tunnel: w573 -> [w591]
                  tunnel: w572 -> [w604]
                  tunnel: w571 -> [w603]
                  tunnel: [w605] -> w570
                  tunnel: w566 -> [w601]
                  tunnel: w565 -> [w600]
                  tunnel: [w599] -> w564
                  tunnel: w562 -> [w598]
                  tunnel: w563 -> [w597]
                  tunnel: w562 -> [w596]
                  tunnel: w561 -> [w595]
                  tunnel: [w594] -> w560
                  tunnel: [w590] -> w556
                  tunnel: w555 -> [w590]
                  tunnel: [w589] -> w554
                  tunnel: w553 -> [w589]
                  tunnel: [w636] -> w574
                  tunnel: w570 -> [w636]
                  tunnel: [w635] -> w569
                  tunnel: [w634] -> w568
                  tunnel: w556 -> [w635]
                  tunnel: w554 -> [w634]
                  frame #0 {
                    n449 = local read "Step Delay (s)"() -> (w576:dbl)
                    n450 = Multiply(x=1000.0, y=w576) -> (x*y=w578:dbl)
                    n451 = Wait (ms)(milliseconds to wait=w578) -> ()  [unwired: 1 out]
                  }
                  frame #1 {
                    n452 = local write "Voltage Gate Value"(w581) -> ()
                    n453 = Number To Fractional String(number=w581, precision (6)=i16 4) -> (F-format string=w587:string)  [unwired: 2 in]
                    n454 = Concatenate Strings("WMO" ("write buffer"), w587, "\n" ("write buffer")) -> (w588:string)
                    n455 = VISA Write(VISA resource name=w583, write buffer=w588, error in (no error)=w582) -> (VISA resource name out=w580:refnum<visa-resource-name>, error out=w579:errorcluster)  [unwired: 1 out]
                  }
                  frame #2 {
                    w602 = u16 0 items=["auto / auto", "1 nA / 1.1 V", "10 nA / 11 V", "100 nA / 110 V", "0.001 mA / 110 V", "0.01 mA / 110 V", "0.1 mA / 110 V", "1 mA / 110 V", "10 mA / 110 V", "100 mA / 110 V"] ("source range\nI source / V source (auto:0)")
                    n456 = local read "Integration Time"() -> (w606:dbl)
                    n457 = call "Keith 236 Fixed Level.vi"("GPIB address"=w591, "create/append"=TRUE, "bias level"=0.0, "sweep level"=w607, "source range\nI source / V source (auto:0)"=w602, "error in"=w604, "delay (sec)"=w606, "count"=1) -> ("error out"=w612:T5)
                    n458 = call "Keith 236 Operate/Standby.vi"("source"=TRUE, "error in"=w612, "GPIB address"=w591) -> ("error out"=w593:T5)
                    n459 = call "Keith 236 Send Trigger.vi"("GPIB address"=w591, "error in"=w593) -> ("error out"=w592:T5)
                    n460 = call "Keith 236 Read Measurement.vi"("error in"=w592, "GPIB address"=w591) -> ("error out"=w605:T5, "display"=w613:T6)  [unwired: 2 out]
                    n461 = Fract/Exp String To Number(string=w613) -> (number=w614:T7)  [unwired: 3 in, 1 out]
                    n462 = Index Array(array=w614) -> (element=w615:T8)  [unwired: 1 in]
                    n463 = Unbundle(w615) -> ("source value"=w616:dbl, "measure value"=w617:dbl)  [unwired: 2 out]
                    n464 = case shown="1" w603 {
                      tunnel: w616 -> [w621 w633]
                      tunnel: w617 -> [w620 w624]
                      tunnel: w601 -> [w619 w629]
                      tunnel: w600 -> [_ w631]
                      tunnel: [w619 w630] -> w599
                      tunnel: w598 -> [_ w628]
                      tunnel: w597 -> [_ w627]
                      tunnel: w596 -> [_ w626]
                      tunnel: w595 -> [w618 w625]
                      tunnel: [w618 w622] -> w594
                      frame 0, Default {
                        n465 = local write "Voltage Drain Value"(w621) -> ()
                        n466 = local write "Current Drain Value"(w620) -> ()
                      }
                      frame 1 {
                        n467 = local write "Current Drain Value"(w633) -> ()
                        n468 = local write "Voltage Drain Value"(w624) -> ()
                        n469 = local write "Time Trace"(w624) -> ()
                        n470 = Replace Array Subset(array=w625, new element=w624, index (row)=w627, index (col)=w626) -> (w622:dbl[][])
                        n471 = Replace Array Subset(array=w629, new element=w624, index=w628) -> (w630:dbl[])
                        n472 = Bundle("Array"=w631, w630) -> (w632:cluster{"Array":dbl[], dbl[]})  [unwired: 1 in]
                        n473 = Transpose 2D Array(2D array=w622) -> (transposed array=w623:dbl[][])
                        n474 = local write "Voltage-Current 2D Graph"(w623) -> ()
                        n475 = local write "IV 1D Graph"(w632) -> ()
                      }
                    }
                  }
                  frame #3 {
                  }
                }
                n476 = local read "Stop Measurements"() -> (w567:bool)
              }
              n477 = local write "1D values"(w539) -> ()
            }
            n478 = local write "2D XY array"(w521) -> ()
          }
          frame #2 {
            w637 = TRUE ("1D Data ready")
            w643 = FALSE ("Stop Measurements")
            n479 = call "Keith 236 Operate/Standby.vi"("source"=FALSE, "error in"=w645, "GPIB address"=w644) -> ("error out"=w647:T5)
            n480 = local write "1D Data ready"(w637) -> ()
            n481 = local write "2D Data ready"(w637) -> ()
            n482 = local write "Error SMU"(w647) -> ()
            n483 = local write "Stop Measurements"(w643) -> ()
            n484 = local write "Start IdVg Sweep"(w643) -> ()
            n485 = VISA Write(VISA resource name=w639, write buffer="WMN0\n", error in (no error)=w638) -> (VISA resource name out=w642:refnum<visa-resource-name>, error out=w641:errorcluster)  [unwired: 1 out]
            n486 = local write "Gate resource"(w642) -> ()
            n487 = local write "Error Gate"(w641) -> ()
          }
        }
      }
      frame 9 {
        n488 = flat-sequence {
          tunnel: [w657] -> w655
          tunnel: [w656] -> w652
          tunnel: [w666] -> w651
          tunnel: [w665] -> w650
          tunnel: [w659] -> w649
          tunnel: [w658] -> w648
          tunnel: w655 -> [w704]
          tunnel: [w710] -> w654
          tunnel: [w709] -> w653
          tunnel: w652 -> [w709]
          tunnel: w651 -> [w708]
          tunnel: w650 -> [w707]
          tunnel: w649 -> [w706]
          tunnel: w648 -> [w705]
          tunnel: w654 -> [w761]
          tunnel: w653 -> [w760]
          frame #0 {
            w665 = u16 0 items=["voltage/current", "current/voltage"] ("source/measure (V/I:0)")
            w671 = u16 0 items=["disabled", "2 readings", "4 readings", "8 readings", "16 readings", "32 readings"] ("filter (disabled:0)")
            w673 = u16 1 items=["OFF", "ON"] ("default delay (on:1)")
            w669 = u16 0 items=["auto / auto", "1 nA / 1.1 V", "10 nA / 11 V", "100 nA / 110 V", "0.001 mA / 110 V", "0.01 mA / 110 V", "0.1 mA / 110 V", "1 mA / 110 V", "10 mA / 110 V", "100 mA / 110 V"] ("compliance/\nmeasurement range (auto:0)")
            w670 = u16 1 items=["fast perod", "medium period", "line cycle period @ 50Hz", "line cycle period @ 60Hz"] ("integration time (medium:1)")
            w668 = u16 0 items=["OFF", "ON"] ("suppression (off:0)")
            w667 = u16 0 items=["local", "remote"] ("sense (local:0)")
            w674 = u16 0 items=["auto / auto", "1 nA / 1.1 V", "10 nA / 11 V", "100 nA / 110 V", "0.001 mA / 110 V", "0.01 mA / 110 V", "0.1 mA / 110 V", "1 mA / 110 V", "10 mA / 110 V", "100 mA / 110 V"] ("source range\nI source / V source (auto:0)")
            w672 = u16 1 items=["DC", "sweep"] ("function (DC:0)")
            n489 = local read "OneWay Sweep"() -> (w680:bool)
            n490 = property on="IV 1D Graph" class="XYGraph (strict)"("YScale.Mapping Mode"=u8 1 ("Y Scale.Mapping Mode")) -> ()  [unwired: 2 in, 2 out]
            n491 = case shown="False" w680 {
              tunnel: [w686 w696] -> w657
              tunnel: [w681 w694] -> w659
              frame False {
                n492 = local read "Start Voltage Drain"() -> (w691:dbl)
                n493 = local read "End Voltage Drain"() -> (w690:dbl)
                n494 = Subtract(x=w691, y=w690) -> (x-y=w689:dbl)
                n495 = local read "Step Voltage Drain"() -> (w692:dbl)
                n496 = Absolute Value(x=w689) -> (abs(x)=w688:dbl)
                n497 = Divide(x=w688, y=w692) -> (x/y=w693:dbl)
                n498 = Increment(x=w693) -> (x+1=w687:dbl)
                n499 = Round To Nearest(number=w687) -> (nearest integer value=w685:dbl)
                n500 = call "subVI_RampGenerator.vi"("Number of Positions"=w685, "End  (um)"=w690, "Start  (um)"=w691) -> ("Array"=w683:dbl[])  [unwired: 1 in]
                n501 = Multiply(x=w685, y=2.0) -> (x*y=w681:dbl)
                n502 = Reverse 1D Array(array=w683) -> (reversed array=w682:dbl[])
                n503 = Build Array (concatenate)(w683, w682) -> (w686:dbl[])
              }
              frame True {
                n504 = local read "Start Voltage Drain"() -> (w700:dbl)
                n505 = local read "End Voltage Drain"() -> (w699:dbl)
                n506 = Subtract(x=w700, y=w699) -> (x-y=w698:dbl)
                n507 = local read "Step Voltage Drain"() -> (w701:dbl)
                n508 = Absolute Value(x=w698) -> (abs(x)=w697:dbl)
                n509 = Divide(x=w697, y=w701) -> (x/y=w702:dbl)
                n510 = Increment(x=w702) -> (x+1=w695:dbl)
                n511 = Round To Nearest(number=w695) -> (nearest integer value=w694:dbl)
                n512 = call "subVI_RampGenerator.vi"("Number of Positions"=w694, "End  (um)"=w699, "Start  (um)"=w700) -> ("Array"=w696:dbl[])  [unwired: 1 in]
              }
            }
            n513 = property on="IV 1D Graph" class="XYGraph (strict)"("XScale.NameLbl.Text"="Drain Voltage (V)" ("Y Scale.Name Label.Text")) -> ()  [unwired: 2 in, 2 out]
            n514 = property on="Time Trace" class="WFChart (strict)"("YScale.NameLbl.Text"="Drain Current (A)" ("Y Scale.Name Label.Text")) -> ()  [unwired: 2 in, 2 out]
            n515 = property on="IV 1D Graph" class="XYGraph (strict)"("YScale.NameLbl.Text"="Drain Current (A)" ("Y Scale.Name Label.Text")) -> ()  [unwired: 2 in, 2 out]
            n516 = local read "Compliance Current Drain"() -> (w678:dbl)
            n517 = local read "Compliance Voltage Drain"() -> (w677:dbl)
            n518 = local read "Start Current Drain"() -> (w676:dbl)
            n519 = local read "SMU GPIB address"() -> (w656:string)
            n520 = local read "Integration Time"() -> (w679:dbl)
            n521 = local read "Error SMU"() -> (w675:errorcluster)
            n522 = call "Keith 236 Basic Config.vi"("GPIB address"=w656, "source range\nI source / V source (auto:0)"=w674, "voltage \ncompliance level"=w677, "current \ncompliance level"=w678, "DC delay (sec)"=w679, "source/measure (V/I:0)"=w665, "default delay (on:1)"=w673, "function (DC:0)"=w672, "filter (disabled:0)"=w671, "source level"=w676, "integration time (medium:1)"=w670, "error in"=w675, "compliance/\nmeasurement range (auto:0)"=w669, "suppression (off:0)"=w668, "sense (local:0)"=w667) -> ("error out"=w666:T5)
            n523 = local write "X scale"(w657) -> ()
            n524 = Initialize Array(0.0, w659) -> (w658:dbl[])
          }
          frame #1 {
            n525 = for {
              N: w706 -> [_]
              tunnel: w704 -> [w719] mode=indexing
              tunnel: [w718] -> w710
              tunnel: w709 -> [w717]
              tunnel: w708 -> [w716]
              tunnel: w707 -> [w715]
              tunnel: w704 -> [w712]
              shift-right: [w711] -> w703
              shift-left: w705 -> [w714]
              i -> [w713]
              stop <- w720 stop-if-true
              n526 = flat-sequence {
                tunnel: w719 -> [w736]
                tunnel: [w734] -> w718
                tunnel: w717 -> [w724]
                tunnel: w716 -> [w733]
                tunnel: w715 -> [w732]
                tunnel: w714 -> [w730]
                tunnel: w713 -> [w729]
                tunnel: w712 -> [w728]
                tunnel: [w727] -> w711
                frame #0 {
                  n527 = local read "Step Delay (s)"() -> (w721:dbl)
                  n528 = Multiply(x=1000.0, y=w721) -> (x*y=w723:dbl)
                  n529 = Wait (ms)(milliseconds to wait=w723) -> ()  [unwired: 1 out]
                }
                frame #1 {
                  w731 = u16 0 items=["auto / auto", "1 nA / 1.1 V", "10 nA / 11 V", "100 nA / 110 V", "0.001 mA / 110 V", "0.01 mA / 110 V", "0.1 mA / 110 V", "1 mA / 110 V", "10 mA / 110 V", "100 mA / 110 V"] ("source range\nI source / V source (auto:0)")
                  n530 = local read "Integration Time"() -> (w735:dbl)
                  n531 = call "Keith 236 Fixed Level.vi"("GPIB address"=w724, "create/append"=TRUE, "bias level"=0.0, "sweep level"=w736, "source range\nI source / V source (auto:0)"=w731, "error in"=w733, "delay (sec)"=w735, "count"=1) -> ("error out"=w741:T5)
                  n532 = call "Keith 236 Operate/Standby.vi"("source"=TRUE, "error in"=w741, "GPIB address"=w724) -> ("error out"=w726:T5)
                  n533 = call "Keith 236 Send Trigger.vi"("GPIB address"=w724, "error in"=w726) -> ("error out"=w725:T5)
                  n534 = call "Keith 236 Read Measurement.vi"("error in"=w725, "GPIB address"=w724) -> ("error out"=w734:T5, "display"=w742:T6)  [unwired: 2 out]
                  n535 = Fract/Exp String To Number(string=w742) -> (number=w743:T7)  [unwired: 3 in, 1 out]
                  n536 = Index Array(array=w743) -> (element=w744:T8)  [unwired: 1 in]
                  n537 = Unbundle(w744) -> ("source value"=w745:dbl, "measure value"=w746:dbl)  [unwired: 2 out]
                  n538 = case shown="0, Default" w732 {
                    tunnel: w745 -> [w754 w757]
                    tunnel: w746 -> [w751 w756]
                    tunnel: w730 -> [w749 w755]
                    tunnel: w729 -> [w752 _]
                    tunnel: w728 -> [w750 _]
                    tunnel: [w748 w755] -> w727
                    frame 0, Default {
                      n539 = local write "Voltage Drain Value"(w754) -> ()
                      n540 = local write "Current Drain Value"(w751) -> ()
                      n541 = local write "Time Trace"(w751) -> ()
                      n542 = Replace Array Subset(array=w749, new element=w751, index=w752) -> (w748:dbl[])
                      n543 = Absolute Value(x=w748) -> (abs(x)=w747:dbl[])
                      n544 = Bundle("Array"=w750, w747) -> (w753:cluster{"Array":dbl[], dbl[]})  [unwired: 1 in]
                      n545 = local write "IV 1D Graph"(w753) -> ()
                    }
                    frame 1 {
                      n546 = local write "Current Drain Value"(w757) -> ()
                      n547 = local write "Voltage Drain Value"(w756) -> ()
                    }
                  }
                }
              }
              n548 = local read "Stop Measurements"() -> (w720:bool)
            }
            n549 = local write "1D values"(w703) -> ()
          }
          frame #2 {
            w759 = FALSE ("Stop Measurements")
            n550 = call "Keith 236 Operate/Standby.vi"("source"=FALSE, "error in"=w761, "GPIB address"=w760) -> ("error out"=w763:T5)
            n551 = local write "1D Data ready"(TRUE ("1D Data ready")) -> ()
            n552 = local write "Stop Measurements"(w759) -> ()
            n553 = local write "Start Drain Sweep"(w759) -> ()
            n554 = local write "Error SMU"(w763) -> ()
          }
        }
      }
      frame 10 {
        n555 = flat-sequence {
          tunnel: [w809] -> w778
          tunnel: [w779] -> w777
          tunnel: [w830] -> w776
          tunnel: [w829] -> w775
          tunnel: [w805] -> w772
          tunnel: [w820] -> w771
          tunnel: [w819] -> w770
          tunnel: [w808] -> w769
          tunnel: [w806] -> w768
          tunnel: [w814] -> w765
          tunnel: [w804] -> w764
          tunnel: w778 -> [w867]
          tunnel: [w866] -> w774
          tunnel: [w865] -> w773
          tunnel: w777 -> [w865]
          tunnel: w776 -> [w864]
          tunnel: w775 -> [w863]
          tunnel: w772 -> [w862]
          tunnel: w771 -> [w861]
          tunnel: w770 -> [w860]
          tunnel: w769 -> [w859]
          tunnel: w768 -> [w858]
          tunnel: [w857] -> w767
          tunnel: [w856] -> w766
          tunnel: w765 -> [w855]
          tunnel: w764 -> [w854]
          tunnel: w774 -> [w971]
          tunnel: w773 -> [w970]
          tunnel: w767 -> [w965]
          tunnel: w766 -> [w964]
          frame #0 {
            w811 = "Drain Current (A)" ("Y Scale.Name Label.Text")
            w829 = u16 0 items=["voltage/current", "current/voltage"] ("source/measure (V/I:0)")
            w835 = u16 0 items=["disabled", "2 readings", "4 readings", "8 readings", "16 readings", "32 readings"] ("filter (disabled:0)")
            w837 = u16 1 items=["OFF", "ON"] ("default delay (on:1)")
            w833 = u16 0 items=["auto / auto", "1 nA / 1.1 V", "10 nA / 11 V", "100 nA / 110 V", "0.001 mA / 110 V", "0.01 mA / 110 V", "0.1 mA / 110 V", "1 mA / 110 V", "10 mA / 110 V", "100 mA / 110 V"] ("compliance/\nmeasurement range (auto:0)")
            w834 = u16 1 items=["fast perod", "medium period", "line cycle period @ 50Hz", "line cycle period @ 60Hz"] ("integration time (medium:1)")
            w832 = u16 0 items=["OFF", "ON"] ("suppression (off:0)")
            w831 = u16 0 items=["local", "remote"] ("sense (local:0)")
            w838 = u16 0 items=["auto / auto", "1 nA / 1.1 V", "10 nA / 11 V", "100 nA / 110 V", "0.001 mA / 110 V", "0.01 mA / 110 V", "0.1 mA / 110 V", "1 mA / 110 V", "10 mA / 110 V", "100 mA / 110 V"] ("source range\nI source / V source (auto:0)")
            w836 = u16 1 items=["DC", "sweep"] ("function (DC:0)")
            n556 = local read "Start Voltage Drain"() -> (w784:dbl)
            n557 = local read "End Voltage Drain"() -> (w783:dbl)
            n558 = local read "Start Voltage Gate"() -> (w782:dbl)
            n559 = local read "End Voltage Gate"() -> (w781:dbl)
            n560 = flat-sequence {
              tunnel: [w845] -> w820
              tunnel: [w844] -> w819
              frame #0 {
                n561 = local read "Gate resource"() -> (w848:refnum<visa-resource-name>)
                n562 = local read "Error Gate"() -> (w849:errorcluster)
                n563 = VISA Write(VISA resource name=w848, write buffer="WMO0\n", error in (no error)=w849) -> (VISA resource name out=w851:refnum<visa-resource-name>, error out=w850:errorcluster)  [unwired: 1 out]
                n564 = VISA Write(VISA resource name=w851, write buffer="WMN1\n", error in (no error)=w850) -> (VISA resource name out=w845:refnum<visa-resource-name>, error out=w844:errorcluster)  [unwired: 1 out]
              }
              frame #1 {
                n565 = Wait (ms)(milliseconds to wait=u32 1000) -> ()  [unwired: 1 out]
              }
            }
            n566 = property on="Voltage-Current 2D Graph" class="IntGraph (strict)"("ZScale.Mapping Mode"=u8 0 ("Y Scale.Mapping Mode")) -> ()  [unwired: 2 in, 2 out]
            n567 = property on="IV 1D Graph" class="XYGraph (strict)"("YScale.Mapping Mode"=u8 0 ("Y Scale.Mapping Mode")) -> ()  [unwired: 2 in, 2 out]
            n568 = local read "Step Voltage Drain"() -> (w785:dbl)
            n569 = local read "Step Voltage Gate"() -> (w780:dbl)
            n570 = property on="Voltage-Current 2D Graph" class="IntGraph (strict)"("ZScale.NameLbl.Text"=w811) -> ()  [unwired: 2 in, 2 out]
            n571 = property on="IV 1D Graph" class="XYGraph (strict)"("YScale.NameLbl.Text"=w811) -> ()  [unwired: 2 in, 2 out]
            n572 = property on="IV 1D Graph" class="XYGraph (strict)"("XScale.NameLbl.Text"="Gate Voltage (V)" ("Y Scale.Name Label.Text")) -> ()  [unwired: 2 in, 2 out]
            n573 = property on="Voltage-Current 2D Graph" class="IntGraph (strict)"("XScale.NameLbl.Text"="Gate Voltage (V)" ("Y Scale.Name Label.Text")) -> ()  [unwired: 2 in, 2 out]
            n574 = property on="Voltage-Current 2D Graph" class="IntGraph (strict)"("YScale.NameLbl.Text"="Drain Voltage (V)" ("Y Scale.Name Label.Text")) -> ()  [unwired: 2 in, 2 out]
            n575 = property on="Time Trace" class="WFChart (strict)"("YScale.NameLbl.Text"="Drain Current (A)" ("Y Scale.Name Label.Text")) -> ()  [unwired: 2 in, 2 out]
            n576 = Greater?(x=w783, y=w784) -> (0:w798:bool)
            n577 = Subtract(x=w784, y=w783) -> (x-y=w827:dbl)
            n578 = Greater?(x=w781, y=w782) -> (0:w802:bool)
            n579 = Subtract(x=w782, y=w781) -> (x-y=w822:dbl)
            n580 = Absolute Value(x=w827) -> (abs(x)=w826:dbl)
            n581 = Absolute Value(x=w822) -> (abs(x)=w823:dbl)
            n582 = Divide(x=w785, y=2.0) -> (x/y=w796:dbl)
            n583 = Divide(x=w780, y=2.0) -> (x/y=w797:dbl)
            n584 = Select(t=1.0, s=w798, f=-1.0) -> (s? t:f=w799:dbl)
            n585 = Select(t=1.0, s=w802, f=-1.0) -> (s? t:f=w801:dbl)
            n586 = local read "Compliance Current Drain"() -> (w842:dbl)
            n587 = local read "Compliance Voltage Drain"() -> (w841:dbl)
            n588 = Multiply(x=w799, y=w785) -> (x*y=w800:dbl)
            n589 = Subtract(x=w784, y=w796) -> (x-y=w795:dbl)
            n590 = Divide(x=w826, y=w785) -> (x/y=w828:dbl)
            n591 = Multiply(x=w801, y=w780) -> (x*y=w803:dbl)
            n592 = Subtract(x=w782, y=w797) -> (x-y=w794:dbl)
            n593 = Divide(x=w823, y=w780) -> (x/y=w821:dbl)
            n594 = local read "Start Current Drain"() -> (w840:dbl)
            n595 = local read "SMU GPIB address"() -> (w779:string)
            n596 = local read "Integration Time"() -> (w843:dbl)
            n597 = local read "Error SMU"() -> (w839:errorcluster)
            n598 = Increment(x=w828) -> (x+1=w825:dbl)
            n599 = Increment(x=w821) -> (x+1=w824:dbl)
            n600 = property on="Voltage-Current 2D Graph" class="IntGraph (strict)"("YScale.Offset"=w795, "YScale.Multiplier"=w800, "YScale.Precision"=u8 1 ("Y Scale.Display Format:Precision")) -> ()  [unwired: 2 in, 2 out]
            n601 = property on="Voltage-Current 2D Graph" class="IntGraph (strict)"("XScale.Offset"=w794, "XScale.Multiplier"=w803, "XScale.Precision"=u8 1 ("X Scale.Display Format:Precision")) -> ()  [unwired: 2 in, 2 out]
            n602 = Round To Nearest(number=w825) -> (nearest integer value=w805:dbl)
            n603 = Round To Nearest(number=w824) -> (nearest integer value=w806:dbl)
            n604 = call "Keith 236 Basic Config.vi"("GPIB address"=w779, "source range\nI source / V source (auto:0)"=w838, "voltage \ncompliance level"=w841, "current \ncompliance level"=w842, "DC delay (sec)"=w843, "source/measure (V/I:0)"=w829, "default delay (on:1)"=w837, "function (DC:0)"=w836, "filter (disabled:0)"=w835, "source level"=w840, "integration time (medium:1)"=w834, "error in"=w839, "compliance/\nmeasurement range (auto:0)"=w833, "suppression (off:0)"=w832, "sense (local:0)"=w831) -> ("error out"=w830:T5)
            n605 = call "subVI_RampGenerator.vi"("Number of Positions"=w805, "End  (um)"=w783, "Start  (um)"=w784) -> ("Array"=w809:dbl[])  [unwired: 1 in]
            n606 = call "subVI_RampGenerator.vi"("Number of Positions"=w806, "End  (um)"=w781, "Start  (um)"=w782) -> ("Array"=w808:dbl[])  [unwired: 1 in]
            n607 = local write "Y scale"(w809) -> ()
            n608 = local write "X scale"(w808) -> ()
            n609 = Initialize Array(0.0, w806) -> (w814:dbl[])
            n610 = Initialize Array(0.0 ("element"), w805, w806) -> (w804:dbl[][])
          }
          frame #1 {
            n611 = for {
              N: w862 -> [_]
              tunnel: w867 -> [w884] mode=indexing
              tunnel: [w883] -> w866
              tunnel: w865 -> [w882]
              tunnel: w864 -> [w881]
              tunnel: w863 -> [w880]
              tunnel: w861 -> [w879]
              tunnel: w860 -> [w878]
              tunnel: w859 -> [w873]
              tunnel: w858 -> [w877]
              tunnel: [w876] -> w857
              tunnel: [w875] -> w856
              tunnel: w855 -> [w872]
              shift-right: [w869] -> w853
              shift-left: w854 -> [w870]
              i -> [w868]
              stop <- w874 stop-if-true
              n612 = for {
                N: w877 -> [_]
                tunnel: w884 -> [w903]
                tunnel: w882 -> [w901]
                tunnel: w880 -> [w899]
                shift-right: [w902] -> w883
                shift-left: w881 -> [w900]
                tunnel: w879 -> [w888]
                tunnel: w878 -> [w887]
                tunnel: w873 -> [w889] mode=indexing
                tunnel: [w886] -> w876
                tunnel: [w885] -> w875
                tunnel: [w897] -> w874
                tunnel: w873 -> [w896]
                shift-right: [w894] -> w871
                shift-left: w872 -> [w895]
                shift-right: [w893] -> w869
                shift-left: w870 -> [w892]
                tunnel: w868 -> [w890]
                i -> [w891]
                stop <- w897 stop-if-true
                n613 = flat-sequence {
                  tunnel: w889 -> [w911]
                  tunnel: w888 -> [w910]
                  tunnel: w887 -> [w909]
                  tunnel: [w908] -> w886
                  tunnel: [w907] -> w885
                  tunnel: w903 -> [w933]
                  tunnel: w901 -> [w917]
                  tunnel: w900 -> [w930]
                  tunnel: w899 -> [w929]
                  tunnel: [w931] -> w898
                  tunnel: w896 -> [w927]
                  tunnel: w891 -> [w926]
                  tunnel: w895 -> [w925]
                  tunnel: [w924] -> w894
                  tunnel: [w923] -> w893
                  tunnel: w892 -> [w922]
                  tunnel: w891 -> [w921]
                  tunnel: w890 -> [w920]
                  tunnel: [w962] -> w902
                  tunnel: w898 -> [w962]
                  frame #0 {
                    n614 = local read "Step Delay (s)"() -> (w904:dbl)
                    n615 = Multiply(x=1000.0, y=w904) -> (x*y=w906:dbl)
                    n616 = Wait (ms)(milliseconds to wait=w906) -> ()  [unwired: 1 out]
                  }
                  frame #1 {
                    n617 = local write "Voltage Gate Value"(w911) -> ()
                    n618 = Number To Fractional String(number=w911, precision (6)=i16 4) -> (F-format string=w915:string)  [unwired: 2 in]
                    n619 = Concatenate Strings("WMO" ("write buffer"), w915, "\n" ("write buffer")) -> (w916:string)
                    n620 = VISA Write(VISA resource name=w910, write buffer=w916, error in (no error)=w909) -> (VISA resource name out=w908:refnum<visa-resource-name>, error out=w907:errorcluster)  [unwired: 1 out]
                  }
                  frame #2 {
                    w928 = u16 0 items=["auto / auto", "1 nA / 1.1 V", "10 nA / 11 V", "100 nA / 110 V", "0.001 mA / 110 V", "0.01 mA / 110 V", "0.1 mA / 110 V", "1 mA / 110 V", "10 mA / 110 V", "100 mA / 110 V"] ("source range\nI source / V source (auto:0)")
                    n621 = local read "Integration Time"() -> (w932:dbl)
                    n622 = call "Keith 236 Fixed Level.vi"("GPIB address"=w917, "create/append"=TRUE, "bias level"=0.0, "sweep level"=w933, "source range\nI source / V source (auto:0)"=w928, "error in"=w930, "delay (sec)"=w932, "count"=1) -> ("error out"=w938:T5)
                    n623 = call "Keith 236 Operate/Standby.vi"("source"=TRUE, "error in"=w938, "GPIB address"=w917) -> ("error out"=w919:T5)
                    n624 = call "Keith 236 Send Trigger.vi"("GPIB address"=w917, "error in"=w919) -> ("error out"=w918:T5)
                    n625 = call "Keith 236 Read Measurement.vi"("error in"=w918, "GPIB address"=w917) -> ("error out"=w931:T5, "display"=w939:T6)  [unwired: 2 out]
                    n626 = Fract/Exp String To Number(string=w939) -> (number=w940:T7)  [unwired: 3 in, 1 out]
                    n627 = Index Array(array=w940) -> (element=w941:T8)  [unwired: 1 in]
                    n628 = Unbundle(w941) -> ("source value"=w942:dbl, "measure value"=w943:dbl)  [unwired: 2 out]
                    n629 = case shown="0, Default" w929 {
                      tunnel: w942 -> [w957 w961]
                      tunnel: w943 -> [w951 w960]
                      tunnel: w927 -> [w955 _]
                      tunnel: w926 -> [w954 _]
                      tunnel: w925 -> [w953 w959]
                      tunnel: [w947 w959] -> w924
                      tunnel: [w946 w958] -> w923
                      tunnel: w922 -> [w952 w958]
                      tunnel: w921 -> [w950 _]
                      tunnel: w920 -> [w949 _]
                      frame 0, Default {
                        n630 = local write "Voltage Drain Value"(w957) -> ()
                        n631 = local write "Current Drain Value"(w951) -> ()
                        n632 = local write "Time Trace"(w951) -> ()
                        n633 = Replace Array Subset(array=w952, new element=w951, index (row)=w949, index (col)=w950) -> (w946:dbl[][])
                        n634 = Replace Array Subset(array=w953, new element=w951, index=w954) -> (w947:dbl[])
                        n635 = Absolute Value(x=w947) -> (abs(x)=w948:dbl[])
                        n636 = Bundle("Array"=w955, w948) -> (w956:cluster{"Array":dbl[], dbl[]})  [unwired: 1 in]
                        n637 = Transpose 2D Array(2D array=w946) -> (transposed array=w945:dbl[][])
                        n638 = Absolute Value(x=w945) -> (abs(x)=w944:dbl[][])
                        n639 = local write "IV 1D Graph"(w956) -> ()
                        n640 = local write "Voltage-Current 2D Graph"(w944) -> ()
                      }
                      frame 1 {
                        n641 = local write "Current Drain Value"(w961) -> ()
                        n642 = local write "Voltage Drain Value"(w960) -> ()
                      }
                    }
                  }
                  frame #3 {
                  }
                }
                n643 = local read "Stop Measurements"() -> (w897:bool)
              }
              n644 = local write "1D values"(w871) -> ()
            }
            n645 = local write "2D XY array"(w853) -> ()
          }
          frame #2 {
            w963 = TRUE ("1D Data ready")
            w969 = FALSE ("Stop Measurements")
            n646 = call "Keith 236 Operate/Standby.vi"("source"=FALSE, "error in"=w971, "GPIB address"=w970) -> ("error out"=w973:T5)
            n647 = local write "1D Data ready"(w963) -> ()
            n648 = local write "2D Data ready"(w963) -> ()
            n649 = local write "Error SMU"(w973) -> ()
            n650 = local write "Stop Measurements"(w969) -> ()
            n651 = local write "Start VdVg Sweep"(w969) -> ()
            n652 = VISA Write(VISA resource name=w965, write buffer="WMN0\n", error in (no error)=w964) -> (VISA resource name out=w968:refnum<visa-resource-name>, error out=w967:errorcluster)  [unwired: 1 out]
            n653 = local write "Gate resource"(w968) -> ()
            n654 = local write "Error Gate"(w967) -> ()
          }
        }
      }
    }
  }
  n655 = Initialize Array(0.0, w8, w8) -> (→"2D XY array":dbl[][])
  n656 = local write "Stop Measurements"(w10) -> ()
  n657 = call "subVI_RampGenerator.vi"("Number of Positions"=u16 1, "End  (um)"=10.0, "Start  (um)"=0.0) -> ("Array"=→"X scale" →"Y scale" →"1D values":dbl[])  [unwired: 1 in]
  "Gate Device Ready" <- w10
  "Error Gate" <- w1
  "Error Current" <- w1
  "Drain Device Ready" <- FALSE ("Drain Device Ready")
  "SMU Device Ready" <- w10
  "Error SMU" <- w1
  "2D Data ready" <- w2
  "1D Data ready" <- w2
